vi "RandomLaser-1-1.vi"() -> ()   [LabVIEW 2014]
doc: "Random Laser Project\nAndré Romero - 2020\nandretec@ifsc.usp.br\n\nMain Program"
uses:
  OceanOptics.ctl
  GlobalVariables.vi
  <vilib>/Analysis/NI_AAL_SigProc.lvlib
  PowerMeterSteps.ctl
  <vilib>/Analysis/NI_AALBase.lvlib
  RL-Signal.ctl
  <vilib>/Utility/file.llb/Write To Spreadsheet File (DBL).vi
  <vilib>/Analysis/2dsp.llb/Integral Method.ctl
  <vilib>/Analysis/NI_AALPro.lvlib
  <vilib>/Analysis/8numeric.llb/1D Numeric Integration.vi
panel:
  out "Time Stamp":string="0:01:34"
  out "array of delay (ms)":u32[](array[numeric])=[842, 1108, 1021, 480, 726, 1312, 337, 999, 437, 1394, 1475, 822, 559, 616, 658, 1372, 991, 596, 810, 891, 815, 681, 1513, 577, 789, 631, 803, 488, 1470, 1213, 1450, 749, 1550, 888, 468, 582, 1321, 1466, 836, 595, 723, 733, 1457, 768, 669, 1441, 1356, 658, 1400, 1611, 522, 560, 750, 650, 906, 623, 657, 1594, 565, 802, 980, 736, 879, 514, 829, 685, 842, 615, 791, 1301, 1389, 1499, 389, 859, 1201, 1412, 555, 678, 866, 605, 785, 914, 554, 703, 796, 663, 608, 1407, 608, 816, 1001, 499, 881, 686, 1365, 829, 700, 715, 728, 1156, 922, 602, 1328, 1888]
  out "delta WL":dbl=0.38690207279938704
  in  "Stop":bool
  out "size(s)":i32=105
  out "Waveform Graph 2":dbl[](graph)=[-1.0602626e-05, -1.8573209307692306e-05, -1.2360805192307691e-05, -7.52886973076923e-06, 1.7781546653846153e-05, 2.90088355e-05, 7.443762192307693e-05, 0.00010577740999999999, 0.00011369514192307692, 0.0001716017673076923, 0.0001952365403846154, 0.00020954966423076922, 0.0002917340261538461, 0.00031620668153846155, 0.00033834876384615384, 0.00035088591038461535, 0.00036754105307692305, 0.0004927123461538461, 0.0005941180961538462, 0.0006408687538461539, 0.0007478033923076922, 0.0008147488615384615, 0.0008696404192307692, 0.0008872695615384616, 0.0009365023846153847, 0.001030977223076923, 0.0013047827038461537, 0.0015105027923076923, 0.0016743372076923077, 0.0017111218769230768, 0.0018390295192307693, 0.0019388902461538462, 0.0019474161, 0.0019474161, 0.001959032780769231, 0.0023469584115384614, 0.002392628811538462, 0.002490708273076923, 0.0025502076961538465, 0.0026105925461538462, 0.0027505951807692305, 0.0028934302884615383, 0.0031883340307692306, 0.003340183265384615, 0.003531661842307692, 0.003809862, 0.004016680999999999, 0.004217133384615384, 0.004234585384615385, 0.004321589269230769, 0.0046734980384615385, 0.0047475690769230765, 0.004773726692307693, 0.004844272115384615, 0.0048776663076923075, 0.004990282038461538, 0.005060921961538461, 0.005060921961538461, 0.0055383183461538464, 0.0056066344230769226, 0.0056979792692307685, 0.0058101301923076925, 0.006037626346153846, 0.006264335346153846, 0.006264335346153846, 0.006384484884615385, 0.006694922461538462, 0.006785941346153846, 0.006852017346153845, 0.007037507692307692, 0.007274539153846154, 0.007666755807692308, 0.007813228653846153, 0.007889473538461539, 0.007837736769230769, 0.007881207153846154, 0.007837807499999998, 0.007895348038461538, 0.008558267, 0.008670603307692306, 0.008750500961538461, 0.008750500961538461, 0.008761567576923077, 0.008665184615384614, 0.008665184615384614, 0.008836726192307692, 0.008947153307692307, 0.009076968, 0.0091185865, 0.009199394846153846, 0.009195958807692308, 0.009228286423076923, 0.009228286423076923, 0.009355492576923077, 0.009418467884615384, 0.009475817653846154, 0.009609611076923076, 0.009646632076923076, 0.009646632076923076, 0.009709267076923076, 0.009727449384615384, 0.009765767038461538, 0.009825513153846152, 0.009825513153846152, 0.009828276692307692]
  out "Motor Target":i32
  out "step error":dbl=4.630004747377598
  out "Numeric Control":i32=571
  out "appended array":dbl[](array[numeric])=[0.006088400884615384, 0.006019662115384615, 0.006051416192307692, 0.006051416192307692, 0.006124910076923076, 0.006172556192307692, 0.006457423115384615, 0.006457423115384615, 0.006727457423076923, 0.006873657153846154, 0.006931027961538462, 0.007085490076923076, 0.007085490076923076, 0.0074338476923076924, 0.0074338476923076924, 0.007682742307692307, 0.0077406902692307685, 0.007894204461538462, 0.008228431961538461, 0.008252353499999998, 0.008392664423076924, 0.008392664423076924, 0.00844546326923077, 0.008496700307692307, 0.008698614653846153, 0.008752471038461537, 0.008752471038461537, 0.008816909615384616, 0.008909836807692306, 0.009049831615384614, 0.009202393884615384, 0.009148910884615384, 0.009148910884615384, 0.00914061496153846, 0.009268187346153846, 0.009268187346153846, 0.009387016038461538, 0.009557217038461538, 0.009557217038461538, 0.009661707846153845, 0.009897883192307692, 0.009843781423076922, 0.010035894461538462, 0.010035894461538462, 0.010075476576923077, 0.009985933461538461, 0.009985933461538461, 0.010022820115384615, 0.009880154038461538, 0.009880154038461538, 0.009872941653846152, 0.009776705576923077, 0.009722396961538461, 0.009722396961538461, 0.00970868323076923, 0.009762843192307693, 0.009601696653846154, 0.009404687, 0.009404687, 0.009369634346153845, 0.009404875038461538, 0.009404875038461538, 0.009498904615384616, 0.009371503269230768, 0.00918766646153846, 0.009124002499999999, 0.009124002499999999, 0.008958641692307694, 0.008990724846153847, 0.00885226673076923, 0.008834460576923076, 0.008834460576923076, 0.008653751769230769, 0.00856737246153846, 0.00856737246153846, 0.008425105807692308, 0.008425105807692308, 0.008219209192307692, 0.008219209192307692, 0.00784359423076923, 0.00784359423076923, 0.007704991961538461, 0.007290269076923077, 0.007167071692307693, 0.007167071692307693, 0.007004637807692307, 0.006663415999999999, 0.006663415999999999, 0.006437745346153846, 0.006437745346153846, 0.006332175461538462, 0.006191508153846154, 0.005999933307692308, 0.005999933307692308, 0.005755351423076923, 0.005602332884615384, 0.005341360192307692, 0.005145278269230769, 0.005095772230769231, 0.005095772230769231, 0.004993629423076923, 0.004931614538461538, 0.004852756999999999, 0.0045647115, 0.004118548884615384, 0.004118548884615384, 0.0038448551038461534, 0.0038448551038461534, 0.0036742806846153846, 0.0035786020692307693, 0.0034039533384615387, 0.003279750280769231, 0.0031362856346153845, 0.002992311446153846, 0.00278225455, 0.00278225455, 0.0027080816499999998, 0.0023620212076923075, 0.0023620212076923075, 0.0022386317153846153, 0.002112930703846154, 0.001966992230769231, 0.001864995396153846, 0.0016025416423076924, 0.0015336607115384615, 0.0015336607115384615, 0.00138643115, 0.001199871676923077, 0.001054965946153846, 0.0009808228153846154, 0.0009352345230769231, 0.0009352345230769231, 0.0008112675961538462, 0.0007670655923076923, 0.0006205916653846153, 0.0005729669423076923, 0.0004712719461538462, 0.0004253776961538461, 0.00037583648423076925, 0.0003179948042307692, 0.0003179948042307692, 0.00023497789076923074, 0.00016738367076923075, 0.00010301030038461539, 0.00010301030038461539, -5.387276884615384e-06, -1.463806623076923e-05, -1.463806623076923e-05, -4.7211138846153846e-05, -6.807878461538462e-05, -6.807878461538462e-05, -7.410832192307692e-05, -7.496382769230768e-05, -7.496382769230768e-05, -7.545941807692307e-05, -5.749450153846154e-05, -5.749450153846154e-05, -3.4196017846153845e-05, -3.935870692307692e-06, 1.5409708653846153e-05, 1.5409708653846153e-05, 6.494484076923077e-05, 0.00010907543384615385, 0.00018819801653846153, 0.00018819801653846153, 0.0002518573846153846, 0.0002518573846153846, 0.00036352903423076923, 0.00036352903423076923, 0.00041147177307692307, 0.0006472696384615385, 0.0007086754153846153, 0.0007086754153846153, 0.0008853873846153846, 0.0008853873846153846, 0.0010021450653846153, 0.0011826555307692308, 0.0011826555307692308, 0.0012722923076923078, 0.0014195047423076923, 0.0014195047423076923, 0.001521211773076923, 0.0019048786115384614, 0.0019904611115384614, 0.0019904611115384614, 0.0022153737230769226, 0.002316673857692308, 0.0024764594846153846, 0.002645395580769231, 0.002645395580769231, 0.0027565079615384618, 0.0028778550384615386, 0.0029616142961538462, 0.0030646022269230767, 0.0033371978846153845, 0.0036325316884615387, 0.003766581919230769, 0.0038838421538461535, 0.004069579192307693, 0.004069579192307693, 0.004217383230769231, 0.004395655846153846, 0.004597885384615385, 0.004702704384615384, 0.005098710807692307, 0.005098710807692307, 0.005233906153846154, 0.005420664076923077, 0.005420664076923077, 0.005705798807692308, 0.005807721769230769, 0.005997826192307692, 0.005997826192307692, 0.006048182961538462, 0.006420420961538461, 0.006442509, 0.006442509, 0.006588312, 0.006697340769230769, 0.0068355065, 0.007070677538461538, 0.007342427192307692, 0.007342427192307692, 0.007521121115384615, 0.0075672636923076915, 0.0075672636923076915, 0.007820148192307693, 0.007926758653846153, 0.008071146807692308, 0.008098770346153847, 0.008098770346153847, 0.008299234846153846, 0.008456086615384615, 0.008540288884615384, 0.008588171423076923, 0.008658632230769231, 0.008842661576923077, 0.008987104346153846, 0.009063884730769231, 0.009099668115384615, 0.009163529076923077, 0.009163529076923077, 0.009278776653846153, 0.00929891473076923, 0.009298505461538462, 0.009352490846153846, 0.009341272000000001, 0.009346393384615384, 0.009460399769230769, 0.009600639961538461, 0.009552550576923077, 0.009686249999999999, 0.009748534884615384, 0.009748534884615384, 0.009754034153846153, 0.009697521692307691, 0.009786861499999999, 0.009818387653846154, 0.009818387653846154, 0.009936413961538462, 0.009839843884615385, 0.009827076692307693, 0.009686187307692308, 0.009518681769230769, 0.009597393769230769, 0.009587433076923077, 0.009642559307692306, 0.009593832346153845, 0.009555409, 0.009555409, 0.009464713423076922, 0.00935705523076923, 0.009246092615384616, 0.009100211692307692, 0.008999765846153846, 0.009005339461538461, 0.00912219803846154, 0.009071167846153846, 0.00880848026923077, 0.008668077115384617, 0.00842139573076923, 0.008434145, 0.00836997776923077, 0.008148135846153846, 0.0079498895, 0.007826445384615384, 0.007592567884615384, 0.007468364384615384, 0.007434496923076923, 0.007345466961538461, 0.0072643729615384615, 0.007099095884615384, 0.006919479576923077, 0.0067396438846153844, 0.006546222961538461, 0.006338919499999999, 0.006158986615384615, 0.0060612904615384615, 0.006015968615384616, 0.006006780769230769, 0.0057571594615384615, 0.005552136384615384, 0.005526767269230769, 0.005398911, 0.005002913961538461, 0.004812826576923077, 0.0045138299230769235, 0.004511429538461538, 0.004511429538461538, 0.00449410023076923, 0.0041596291538461535, 0.003989496653846154, 0.003923653961538461, 0.0038588970384615382, 0.00366277415, 0.00366277415, 0.003438994126923077, 0.003438994126923077, 0.0033308669038461538, 0.002999190473076923, 0.002931602423076923, 0.002931602423076923, 0.0028267784884615384, 0.0024557568115384613, 0.0024557568115384613, 0.0023362327538461536, 0.0020663858423076924, 0.001972159503846154, 0.001749807696153846, 0.0017157880038461539, 0.0014433754807692306, 0.0013448947230769231, 0.0013372903384615386, 0.001248845923076923, 0.0010909017884615383, 0.0009248163, 0.0007581637961538461, 0.000743720346153846, 0.00072130105, 0.0006646627576923077, 0.0005633626769230768, 0.0005633626769230768, 0.0004006925538461538, 0.0003739367319230769, 0.00025180435423076923, 0.0002452021223076923, 0.00022705456884615383, 0.00016810932153846155, 8.971818923076923e-05, 7.203049038461537e-05, 6.765868923076923e-05, 4.472013076923077e-05, 1.969299146153846e-05, 5.592379307692308e-06, 5.232428384615384e-06, 2.3887723115384613e-06, -7.4403199230769226e-06, -1.0602626e-05, -1.8573209307692306e-05, -1.2360805192307691e-05, -7.52886973076923e-06, 1.7781546653846153e-05, 2.90088355e-05, 7.443762192307693e-05, 0.00010577740999999999, 0.00011369514192307692, 0.0001716017673076923, 0.0001952365403846154, 0.00020954966423076922, 0.0002917340261538461, 0.00031620668153846155, 0.00033834876384615384, 0.00035088591038461535, 0.00036754105307692305, 0.0004927123461538461, 0.0005941180961538462, 0.0006408687538461539, 0.0007478033923076922, 0.0008147488615384615, 0.0008696404192307692, 0.0008872695615384616, 0.0009365023846153847, 0.001030977223076923, 0.0013047827038461537, 0.0015105027923076923, 0.0016743372076923077, 0.0017111218769230768, 0.0018390295192307693, 0.0019388902461538462, 0.0019474161, 0.0019474161, 0.001959032780769231, 0.0023469584115384614, 0.002392628811538462, 0.002490708273076923, 0.0025502076961538465, 0.0026105925461538462, 0.0027505951807692305, 0.0028934302884615383, 0.0031883340307692306, 0.003340183265384615, 0.003531661842307692, 0.003809862, 0.004016680999999999, 0.004217133384615384, 0.004234585384615385, 0.004321589269230769, 0.0046734980384615385, 0.0047475690769230765, 0.004773726692307693, 0.004844272115384615, 0.0048776663076923075, 0.004990282038461538, 0.005060921961538461, 0.005060921961538461, 0.0055383183461538464, 0.0056066344230769226, 0.0056979792692307685, 0.0058101301923076925, 0.006037626346153846, 0.006264335346153846, 0.006264335346153846, 0.006384484884615385, 0.006694922461538462, 0.006785941346153846, 0.006852017346153845, 0.007037507692307692, 0.007274539153846154, 0.007666755807692308, 0.007813228653846153, 0.007889473538461539, 0.007837736769230769, 0.007881207153846154, 0.007837807499999998, 0.007895348038461538, 0.008558267, 0.008670603307692306, 0.008750500961538461, 0.008750500961538461, 0.008761567576923077, 0.008665184615384614, 0.008665184615384614, 0.008836726192307692, 0.008947153307692307, 0.009076968, 0.0091185865, 0.009199394846153846, 0.009195958807692308, 0.009228286423076923, 0.009228286423076923, 0.009355492576923077, 0.009418467884615384, 0.009475817653846154, 0.009609611076923076, 0.009646632076923076, 0.009646632076923076, 0.009709267076923076, 0.009727449384615384, 0.009765767038461538, 0.009825513153846152, 0.009825513153846152, 0.009828276692307692, 0.009801360576923077, 0.009814088346153845, 0.00984271126923077, 0.009860809384615385, 0.009873510307692308, 0.0098137955, 0.009603421384615384, 0.009603421384615384, 0.00955146523076923, 0.00949282146153846, 0.009467082038461538, 0.009361033923076922, 0.00934043826923077, 0.009350373884615385, 0.009290900884615384, 0.009237378461538461, 0.009179430499999999, 0.00911498746153846, 0.009004738576923075, 0.008925467807692307, 0.008768998461538462, 0.008696039153846154, 0.008603960038461539, 0.008526891307692307, 0.008526891307692307, 0.008431125346153846, 0.008406236653846154, 0.008305084269230769, 0.008305084269230769, 0.007906728076923077, 0.007751959269230769, 0.007706900269230769, 0.0076030416923076926, 0.007524473884615385, 0.007239447076923077, 0.007210126076923076, 0.00707238573076923, 0.006996408615384615, 0.006782788269230768, 0.006661043807692307, 0.006556346153846154, 0.006556346153846154, 0.006124177538461538, 0.006010642153846154, 0.005964971538461539, 0.005829333346153846, 0.005684320153846154, 0.005567964846153846, 0.005567964846153846, 0.005230584730769231, 0.005230584730769231, 0.00491325, 0.004761246499999999, 0.0046623946923076915, 0.004590434807692308, 0.004465162961538461, 0.004297437115384615, 0.004162477307692308, 0.004078199769230769, 0.003986143884615385, 0.0038567899230769233, 0.0035312552846153847, 0.003443240823076923, 0.003361292719230769, 0.0032899939346153844, 0.0032048941076923076, 0.0030188552615384614, 0.0029103387192307693, 0.0027534209384615384, 0.0025445671499999996, 0.0024274378884615385, 0.0022463663923076925, 0.002153195626923077, 0.002153195626923077, 0.001970726030769231, 0.0015185043307692307, 0.0014648517576923076, 0.00142660865, 0.0013723234038461537, 0.0013325882807692308, 0.0011872456538461538, 0.0011872456538461538, 0.0009419369653846152, 0.0009419369653846152, 0.0007446580500000001, 0.0005823951846153846, 0.0005605902038461537, 0.0005284770346153846, 0.00048518973461538455, 0.0003851460153846154, 0.00034837271076923075, 0.00029723269115384615, 0.00029723269115384615, 0.0001553477396153846, 0.0001553477396153846, 0.00010404294076923076, 4.2784963846153846e-05, 4.2784963846153846e-05, -7.568358769230769e-05, -8.80733123076923e-05, -8.80733123076923e-05, -0.00011827445499999998, -0.00014029274807692306, -0.00014605101076923076, -0.00014586807653846153, -0.00014213945615384614, -0.00014143732615384615, -0.00013074085692307692, -0.00010745426653846153, -8.991409423076923e-05]
  out "Locations":dbl[](array[numeric])=[152.05783514633893, 357.0837553051094, 566.3699952526224]
  out "Amplitudes":dbl[](array[numeric])=[-7.71015385680156e-05, -1.3525658190277859e-05, -0.0001490156983661843]
  out "standard deviation":dbl=3.0125010126431166 format="%0.2f"
  out "mean":dbl=207.15608005314175 format="%0.2f"
  out "Array":dbl[](array[numeric])=[205.02592015877045, 209.28623994751302]
  out "# found":i32=3
  in  "Select Light Source":u16(ring)=6
  in  "Tab Control":T1(tab)=enum."Aquisition"
  out "Current Step":dbl=103.0
  out "Running":bool=TRUE
  in  "Range List":T2(array[cluster])=[{"Name"="Sample", "Inicial"=500.0, "Final"=700.0}]
  out "Current Position":dbl=104.0
  out "Min power to Aqc":dbl
  out "Max power to Aqc":dbl
  out "Low power":bool
  out "Max power":bool
  in  "Clear Dark Spec":bool caption="Blank Button"
  in  "Average":i32=5
  in  "Integration Time":i32=100
  out "Spectrum":T3(graph)
  in  "Store Dark Spec":bool caption="Blank Button"
  in  "threshold":dbl=300.0 format="%0.2f"
  in  "width":i32=20 min=3
  out "Power Meter [W]":dbl=0.03652572625 format="%#_4p"
  in  "Power up":bool
  in  "Power down":bool
  in  "Half Power":bool
  in  "min Power":bool
  in  "max Power Go":bool
  out "Max Power":dbl=0.010075476576923077 format="%#_3p"
  out "Min Power":dbl=-0.00014605101076923076 format="%#_3p"
  in  "Correct Electrical Dark":bool
  out "table":string[][](table)=[["Name", "FWHM", "Peak", "WL"], ["Sample", "283", "0", "0.00"]]
  out "FWHM":dbl=283.41913100133013 format="%#_4g"
  out "Power Meter":dbl=0.03652572625 format="%#_4p"
  in  "Tuning Motor":bool
  out "Power Meter":dbl(graph)=-8.991409423076923e-05
  out "Min Power":dbl=-0.00014605101076923076 format="%#_3p"
  out "Max Power":dbl=0.010075476576923077 format="%#_3p"
  out "threshold":dbl=0.004964712783076923
  out "Motor Steps Max":i32=104
  out "peak":cluster{dbl[], dbl[]}(graph)={[0.0005015534046874999, 0.0004468511640625, 0.00042210990624999995, 0.0004196072953125, 0.0004832955703125, 0.00061629739375, 0.0006558638234375, 0.0007916550203125, 0.0008665692796875, 0.0009977359703125, 0.0011809348499999999, 0.0014192177328125, 0.0014146657125, 0.001802492625, 0.001933848765625, 0.002189746375, 0.002470051546875, 0.0026339437656249997, 0.002995718203125, 0.0031850202499999996, 0.003397749609375, 0.0038501235468749997, 0.00424369390625, 0.004263668234375, 0.00491242171875, 0.005129561390625001, 0.005458205125, 0.005549518390625, 0.0062437480625, 0.00666187115625, 0.0070897651249999995, 0.007395214921875, 0.00802906796875, 0.008537028765625, 0.00851176228125, 0.008568135671875001, 0.009842375578125, 0.010231534546875, 0.010585043484374999, 0.011054932109375, 0.011588129562499999, 0.012016717671875, 0.0123040546875, 0.013023524656249999, 0.013643318375000001, 0.014436681515624999, 0.01473497978125, 0.014904356796875, 0.0159008428125, 0.016111576406249998, 0.0166677578125, 0.01671055796875, 0.01781797625, 0.018240680156249998, 0.0187542390625, 0.019142343125, 0.0198526453125, 0.01996271609375, 0.02116104, 0.0210028971875, 0.022299682343750002, 0.022769914375000002, 0.02304846125, 0.0231955665625, 0.023897850781249997, 0.024010065, 0.02472973140625, 0.02519956328125, 0.025853811562500002, 0.026471383125, 0.026681425468750002, 0.02802214578125, 0.0278189225, 0.02824113765625, 0.02908268078125, 0.0292354059375, 0.030335440468750002, 0.030317477656249998, 0.03099246828125, 0.03051971140625, 0.031873135625, 0.031079078281250002, 0.032200833125, 0.03170667328125, 0.031286408125, 0.0332111609375, 0.03241316296875, 0.03332632484375, 0.03400264828125, 0.0332313328125, 0.033794730625, 0.03382630828125, 0.03476316046875, 0.034105763125, 0.0363623665625, 0.0356505421875, 0.03637592890625, 0.03534870921875, 0.034879485625, 0.03543325, 0.03644525421875, 0.0360509496875, 0.03622908546875, 0.0367265165625], [0.0, 0.0, 0.0, 0.0, 0.0, 0.0, 0.0, 0.0, 0.0, 0.0, 394.1588118886737, 394.1588118886737, 431.6253969371716, 498.6580958932715, 726.8856416219951, 730.4930041074641, 924.368639084171, 924.368639084171, 1127.8876724584377, 1176.6893948954707, 1257.9781408404046, 1467.6796179824566, 1607.7224288634548, 1607.7224288634548, 1680.7493036733524, 2162.6044383453827, 2162.6044383453827, 2448.692515986958, 2958.1440153813733, 3289.2072493799756, 3712.6227202169744, 3916.1593851910925, 4488.731356999813, 4745.2298607199955, 4745.2298607199955, 5198.759914364481, 6270.088662889236, 6752.182794036469, 6752.182794036469, 7804.8560091986965, 7277.151040936606, 8792.865300035679, 9705.844619862504, 10118.9500660173, 10697.214391856975, 11484.64595778735, 12094.126688665461, 11954.607877343742, 13538.141020872097, 13237.333536906832, 13237.333536906832, 14090.070182374848, 14076.663576921685, 16519.70865370654, 17067.47933725341, 17301.50532254216, 18483.407890232967, 19382.85944297429, 20252.918803668017, 20252.918803668017, 21897.31684455097, 21881.77133506106, 22939.78950340062, 22939.78950340062, 24400.94207257171, 24400.94207257171, 21943.9132770401, 25836.512442775784, 26753.422445361583, 28622.125850531873, 28566.341648867947, 30696.155691767697, 30696.155691767697, 31037.50720247306, 31952.22245683209, 31579.102102413905, 31579.102102413905, 33472.21756510413, 35005.5223676299, 35573.41340181915, 35750.55108838855, 35924.52495802316, 35751.327930291336, 35751.327930291336, 35440.30537928901, 37586.25874441115, 37883.715024127945, 40728.053135189504, 40728.053135189504, 38884.561951946256, 39029.25713331435, 39029.25713331435, 39436.46265344174, 41071.4281739883, 43284.48665620081, 43284.48665620081, 42497.26030199413, 41645.324274929924, 40896.30949743132, 42085.672828850686, 42085.672828850686, 44605.47818116084, 44668.345249601494, 43659.80224543728]}
  out "peak Log":cluster{dbl[], dbl[]}(graph)={[0.0005015534046874999, 0.0004468511640625, 0.00042210990624999995, 0.0004196072953125, 0.0004832955703125, 0.00061629739375, 0.0006558638234375, 0.0007916550203125, 0.0008665692796875, 0.0009977359703125, 0.0011809348499999999, 0.0014192177328125, 0.0014146657125, 0.001802492625, 0.001933848765625, 0.002189746375, 0.002470051546875, 0.0026339437656249997, 0.002995718203125, 0.0031850202499999996, 0.003397749609375, 0.0038501235468749997, 0.00424369390625, 0.004263668234375, 0.00491242171875, 0.005129561390625001, 0.005458205125, 0.005549518390625, 0.0062437480625, 0.00666187115625, 0.0070897651249999995, 0.007395214921875, 0.00802906796875, 0.008537028765625, 0.00851176228125, 0.008568135671875001, 0.009842375578125, 0.010231534546875, 0.010585043484374999, 0.011054932109375, 0.011588129562499999, 0.012016717671875, 0.0123040546875, 0.013023524656249999, 0.013643318375000001, 0.014436681515624999, 0.01473497978125, 0.014904356796875, 0.0159008428125, 0.016111576406249998, 0.0166677578125, 0.01671055796875, 0.01781797625, 0.018240680156249998, 0.0187542390625, 0.019142343125, 0.0198526453125, 0.01996271609375, 0.02116104, 0.0210028971875, 0.022299682343750002, 0.022769914375000002, 0.02304846125, 0.0231955665625, 0.023897850781249997, 0.024010065, 0.02472973140625, 0.02519956328125, 0.025853811562500002, 0.026471383125, 0.026681425468750002, 0.02802214578125, 0.0278189225, 0.02824113765625, 0.02908268078125, 0.0292354059375, 0.030335440468750002, 0.030317477656249998, 0.03099246828125, 0.03051971140625, 0.031873135625, 0.031079078281250002, 0.032200833125, 0.03170667328125, 0.031286408125, 0.0332111609375, 0.03241316296875, 0.03332632484375, 0.03400264828125, 0.0332313328125, 0.033794730625, 0.03382630828125, 0.03476316046875, 0.034105763125, 0.0363623665625, 0.0356505421875, 0.03637592890625, 0.03534870921875, 0.034879485625, 0.03543325, 0.03644525421875, 0.0360509496875, 0.03622908546875, 0.0367265165625], [0.0, 0.0, 0.0, 0.0, 0.0, 0.0, 0.0, 0.0, 0.0, 0.0, 394.1588118886737, 394.1588118886737, 431.6253969371716, 498.6580958932715, 726.8856416219951, 730.4930041074641, 924.368639084171, 924.368639084171, 1127.8876724584377, 1176.6893948954707, 1257.9781408404046, 1467.6796179824566, 1607.7224288634548, 1607.7224288634548, 1680.7493036733524, 2162.6044383453827, 2162.6044383453827, 2448.692515986958, 2958.1440153813733, 3289.2072493799756, 3712.6227202169744, 3916.1593851910925, 4488.731356999813, 4745.2298607199955, 4745.2298607199955, 5198.759914364481, 6270.088662889236, 6752.182794036469, 6752.182794036469, 7804.8560091986965, 7277.151040936606, 8792.865300035679, 9705.844619862504, 10118.9500660173, 10697.214391856975, 11484.64595778735, 12094.126688665461, 11954.607877343742, 13538.141020872097, 13237.333536906832, 13237.333536906832, 14090.070182374848, 14076.663576921685, 16519.70865370654, 17067.47933725341, 17301.50532254216, 18483.407890232967, 19382.85944297429, 20252.918803668017, 20252.918803668017, 21897.31684455097, 21881.77133506106, 22939.78950340062, 22939.78950340062, 24400.94207257171, 24400.94207257171, 21943.9132770401, 25836.512442775784, 26753.422445361583, 28622.125850531873, 28566.341648867947, 30696.155691767697, 30696.155691767697, 31037.50720247306, 31952.22245683209, 31579.102102413905, 31579.102102413905, 33472.21756510413, 35005.5223676299, 35573.41340181915, 35750.55108838855, 35924.52495802316, 35751.327930291336, 35751.327930291336, 35440.30537928901, 37586.25874441115, 37883.715024127945, 40728.053135189504, 40728.053135189504, 38884.561951946256, 39029.25713331435, 39029.25713331435, 39436.46265344174, 41071.4281739883, 43284.48665620081, 43284.48665620081, 42497.26030199413, 41645.324274929924, 40896.30949743132, 42085.672828850686, 42085.672828850686, 44605.47818116084, 44668.345249601494, 43659.80224543728]}
  out "FWHM":cluster{dbl[], dbl[]}(graph)={[0.0005015534046874999, 0.0004468511640625, 0.00042210990624999995, 0.0004196072953125, 0.0004832955703125, 0.00061629739375, 0.0006558638234375, 0.0007916550203125, 0.0008665692796875, 0.0009977359703125, 0.0011809348499999999, 0.0014192177328125, 0.0014146657125, 0.001802492625, 0.001933848765625, 0.002189746375, 0.002470051546875, 0.0026339437656249997, 0.002995718203125, 0.0031850202499999996, 0.003397749609375, 0.0038501235468749997, 0.00424369390625, 0.004263668234375, 0.00491242171875, 0.005129561390625001, 0.005458205125, 0.005549518390625, 0.0062437480625, 0.00666187115625, 0.0070897651249999995, 0.007395214921875, 0.00802906796875, 0.008537028765625, 0.00851176228125, 0.008568135671875001, 0.009842375578125, 0.010231534546875, 0.010585043484374999, 0.011054932109375, 0.011588129562499999, 0.012016717671875, 0.0123040546875, 0.013023524656249999, 0.013643318375000001, 0.014436681515624999, 0.01473497978125, 0.014904356796875, 0.0159008428125, 0.016111576406249998, 0.0166677578125, 0.01671055796875, 0.01781797625, 0.018240680156249998, 0.0187542390625, 0.019142343125, 0.0198526453125, 0.01996271609375, 0.02116104, 0.0210028971875, 0.022299682343750002, 0.022769914375000002, 0.02304846125, 0.0231955665625, 0.023897850781249997, 0.024010065, 0.02472973140625, 0.02519956328125, 0.025853811562500002, 0.026471383125, 0.026681425468750002, 0.02802214578125, 0.0278189225, 0.02824113765625, 0.02908268078125, 0.0292354059375, 0.030335440468750002, 0.030317477656249998, 0.03099246828125, 0.03051971140625, 0.031873135625, 0.031079078281250002, 0.032200833125, 0.03170667328125, 0.031286408125, 0.0332111609375, 0.03241316296875, 0.03332632484375, 0.03400264828125, 0.0332313328125, 0.033794730625, 0.03382630828125, 0.03476316046875, 0.034105763125, 0.0363623665625, 0.0356505421875, 0.03637592890625, 0.03534870921875, 0.034879485625, 0.03543325, 0.03644525421875, 0.0360509496875, 0.03622908546875, 0.0367265165625], [397.83240728192527, 415.17504165662353, 426.25368524810295, 426.25368524810295, 206.73115418767736, 463.69050128006853, 463.69050128006853, 20.243933101369635, 20.243933101369635, 17.116594601847964, 20.241392797112326, 20.241392797112326, 28.609780989435308, 26.179034684086332, 28.5989916901716, 28.949572169655312, 31.723831233679903, 31.723831233679903, 30.6722195921933, 31.723831233679903, 29.98647772865229, 29.632206705867475, 28.588191211899016, 28.588191211899016, 29.28175605364379, 27.533626517494895, 27.533626517494895, 25.442507029580838, 23.695414233195834, 20.560596555511665, 18.812252502514298, 18.462714458332698, 15.671948237431252, 16.368473811981517, 16.368473811981517, 15.322715880405667, 13.578930006455039, 13.578930006455039, 13.578930006455039, 12.882578171121622, 12.533608422419206, 12.533608422419206, 11.488417756278523, 11.488417756278523, 11.488417756278523, 11.488417756278523, 11.140990757941722, 10.792152517895033, 10.792152517895033, 10.792152517895033, 10.792152517895033, 10.792152517895033, 10.792152517895033, 10.095886809932495, 10.095886809932495, 10.443358144362264, 9.74713631806128, 9.74713631806128, 9.74713631806128, 9.74713631806128, 9.74713631806128, 10.095886809932495, 9.74713631806128, 9.74713631806128, 9.74713631806128, 9.74713631806128, 9.74713631806128, 9.74713631806128, 9.398429722999595, 9.050914067624603, 9.398429722999595, 9.399620662686289, 9.399620662686289, 9.74713631806128, 9.74713631806128, 9.74713631806128, 9.74713631806128, 9.398429722999595, 9.050914067624603, 9.050914067624603, 9.050914067624603, 9.399620662686289, 9.74713631806128, 9.74713631806128, 8.702251384519855, 9.398429722999595, 9.398429722999595, 9.050914067624603, 9.050914067624603, 9.050914067624603, 9.050914067624603, 9.050914067624603, 9.74713631806128, 9.399620662686289, 9.399620662686289, 9.399620662686289, 9.050914067624603, 9.050914067624603, 9.050914067624603, 9.399620662686289, 9.399620662686289, 9.050914067624603, 9.050914067624603, 9.74713631806128]}
  in  "File name":string="N28-TiO2-30uL-2"
  out "Current Step":dbl=104.0
  out "Power Meter [W]":dbl=0.03652572625 format="%#_4p"
  out "Running":bool
  in  "Step Stop":i32=104
  in  "Save Aquisition":bool
  in  "Play Aquisition":bool
  out "Integration":cluster{dbl[], dbl[]}(graph)={[0.0005015534046874999, 0.0004468511640625, 0.00042210990624999995, 0.0004196072953125, 0.0004832955703125, 0.00061629739375, 0.0006558638234375, 0.0007916550203125, 0.0008665692796875, 0.0009977359703125, 0.0011809348499999999, 0.0014192177328125, 0.0014146657125, 0.001802492625, 0.001933848765625, 0.002189746375, 0.002470051546875, 0.0026339437656249997, 0.002995718203125, 0.0031850202499999996, 0.003397749609375, 0.0038501235468749997, 0.00424369390625, 0.004263668234375, 0.00491242171875, 0.005129561390625001, 0.005458205125, 0.005549518390625, 0.0062437480625, 0.00666187115625, 0.0070897651249999995, 0.007395214921875, 0.00802906796875, 0.008537028765625, 0.00851176228125, 0.008568135671875001, 0.009842375578125, 0.010231534546875, 0.010585043484374999, 0.011054932109375, 0.011588129562499999, 0.012016717671875, 0.0123040546875, 0.013023524656249999, 0.013643318375000001, 0.014436681515624999, 0.01473497978125, 0.014904356796875, 0.0159008428125, 0.016111576406249998, 0.0166677578125, 0.01671055796875, 0.01781797625, 0.018240680156249998, 0.0187542390625, 0.019142343125, 0.0198526453125, 0.01996271609375, 0.02116104, 0.0210028971875, 0.022299682343750002, 0.022769914375000002, 0.02304846125, 0.0231955665625, 0.023897850781249997, 0.024010065, 0.02472973140625, 0.02519956328125, 0.025853811562500002, 0.026471383125, 0.026681425468750002, 0.02802214578125, 0.0278189225, 0.02824113765625, 0.02908268078125, 0.0292354059375, 0.030335440468750002, 0.030317477656249998, 0.03099246828125, 0.03051971140625, 0.031873135625, 0.031079078281250002, 0.032200833125, 0.03170667328125, 0.031286408125, 0.0332111609375, 0.03241316296875, 0.03332632484375, 0.03400264828125, 0.0332313328125, 0.033794730625, 0.03382630828125, 0.03476316046875, 0.034105763125, 0.0363623665625, 0.0356505421875, 0.03637592890625, 0.03534870921875, 0.034879485625, 0.03543325, 0.03644525421875, 0.0360509496875, 0.03622908546875, 0.0367265165625], [0.0, 0.0, 0.0, 0.0, 0.0, 0.0, 0.0, 0.0, 0.0, 0.0, 394.1588118886737, 394.1588118886737, 431.6253969371716, 498.6580958932715, 726.8856416219951, 730.4930041074641, 924.368639084171, 924.368639084171, 1127.8876724584377, 1176.6893948954707, 1257.9781408404046, 1467.6796179824566, 1607.7224288634548, 1607.7224288634548, 1680.7493036733524, 2162.6044383453827, 2162.6044383453827, 2448.692515986958, 2958.1440153813733, 3289.2072493799756, 3712.6227202169744, 3916.1593851910925, 4488.731356999813, 4745.2298607199955, 4745.2298607199955, 5198.759914364481, 6270.088662889236, 6752.182794036469, 6752.182794036469, 7804.8560091986965, 7277.151040936606, 8792.865300035679, 9705.844619862504, 10118.9500660173, 10697.214391856975, 11484.64595778735, 12094.126688665461, 11954.607877343742, 13538.141020872097, 13237.333536906832, 13237.333536906832, 14090.070182374848, 14076.663576921685, 16519.70865370654, 17067.47933725341, 17301.50532254216, 18483.407890232967, 19382.85944297429, 20252.918803668017, 20252.918803668017, 21897.31684455097, 21881.77133506106, 22939.78950340062, 22939.78950340062, 24400.94207257171, 24400.94207257171, 21943.9132770401, 25836.512442775784, 26753.422445361583, 28622.125850531873, 28566.341648867947, 30696.155691767697, 30696.155691767697, 31037.50720247306, 31952.22245683209, 31579.102102413905, 31579.102102413905, 33472.21756510413, 35005.5223676299, 35573.41340181915, 35750.55108838855, 35924.52495802316, 35751.327930291336, 35751.327930291336, 35440.30537928901, 37586.25874441115, 37883.715024127945, 40728.053135189504, 40728.053135189504, 38884.561951946256, 39029.25713331435, 39029.25713331435, 39436.46265344174, 41071.4281739883, 43284.48665620081, 43284.48665620081, 42497.26030199413, 41645.324274929924, 40896.30949743132, 42085.672828850686, 42085.672828850686, 44605.47818116084, 44668.345249601494, 43659.80224543728]}
  in  "correction factor":dbl=0.64
  out "Power Value":dbl=0.03652572625 caption="Optical Power [W]" format="%#_4p"
  in  "Average Time (0.0)":dbl=0.05
  out "P Meter Delay (ms)":u32=106
  out "Spectrum delay (ms)":u32=707
  out "Delayreturn":u32
  # "Set power to Aquisition"
  # "Move Step Motor"
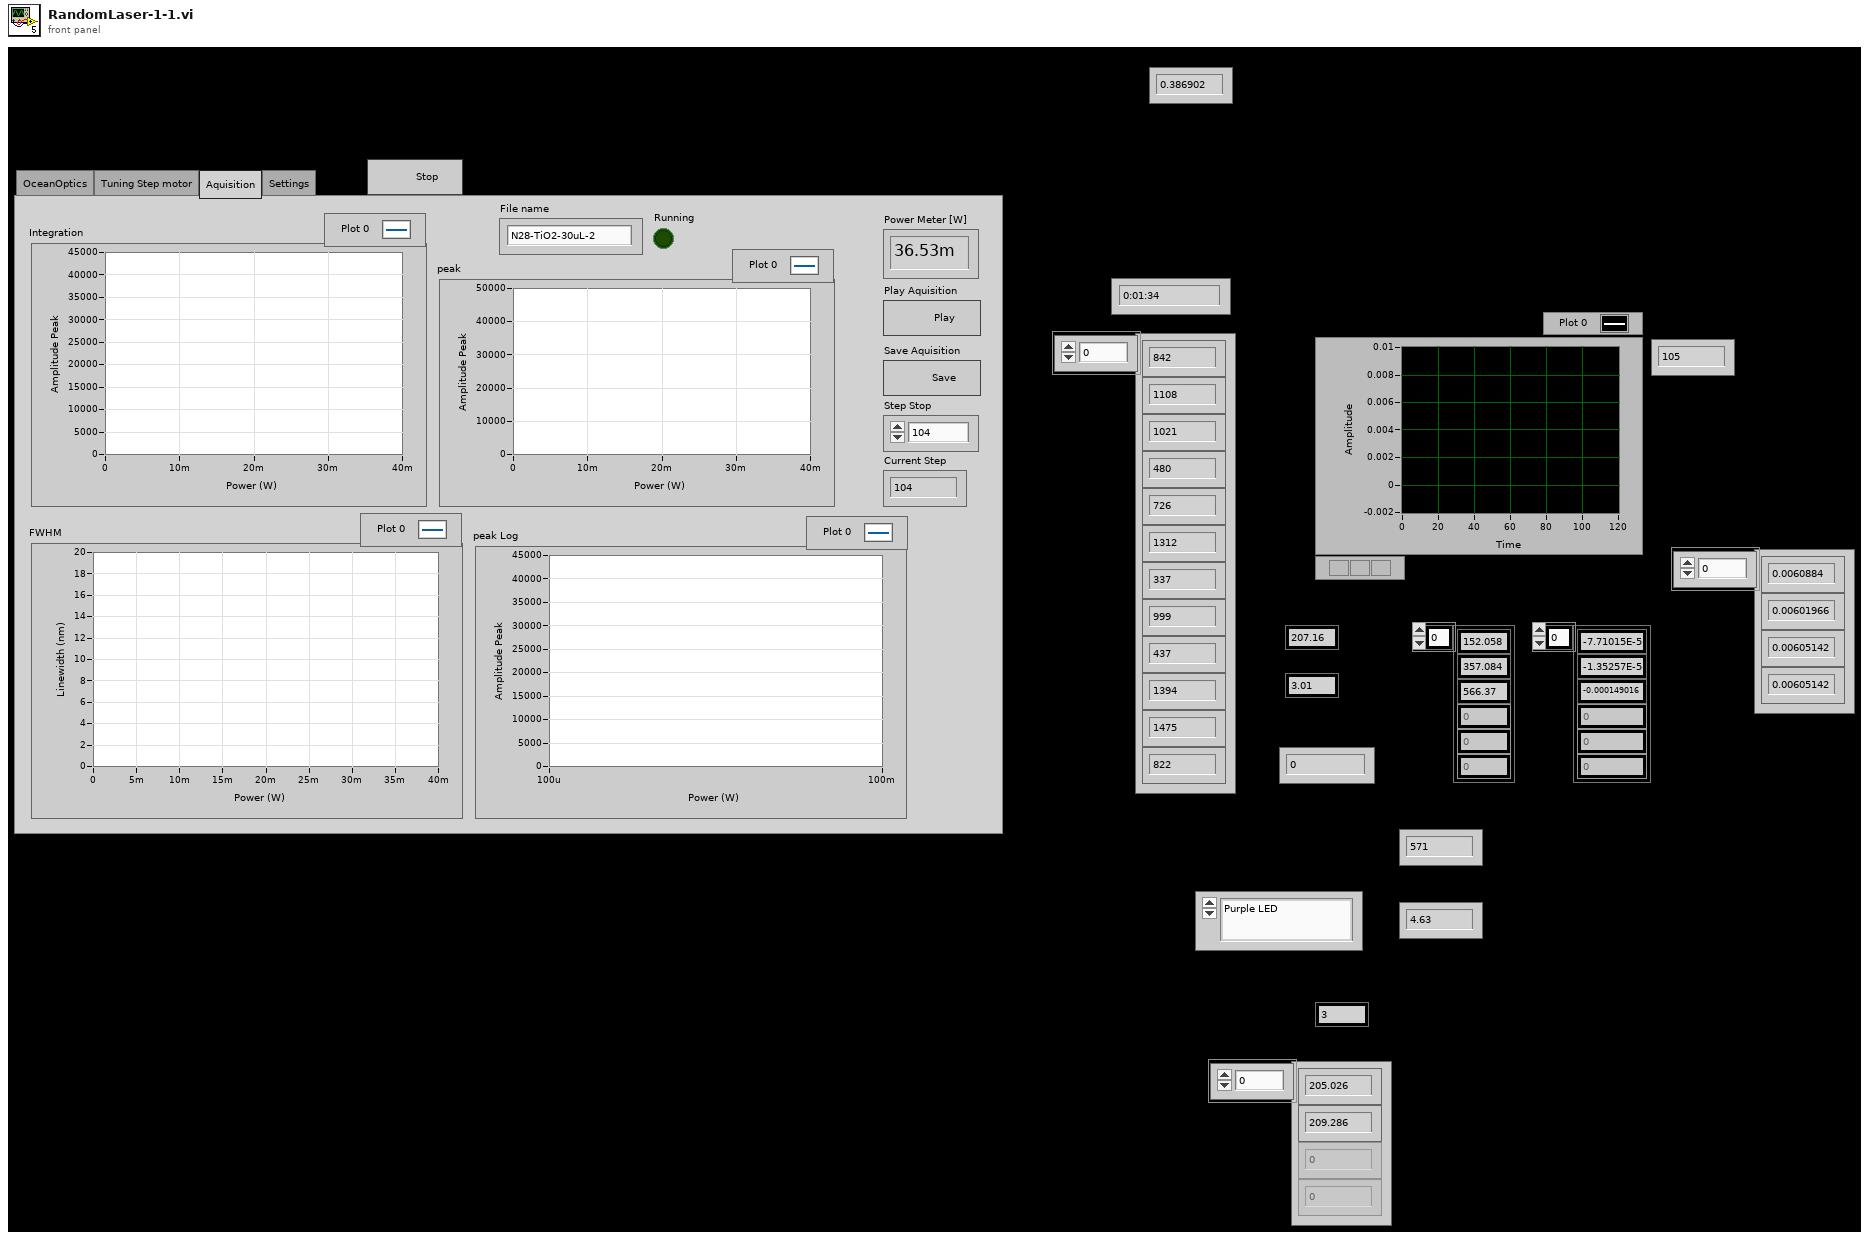
[diagram p1: front panel]
types:
  T1 = enum32{"OceanOptics", "Tuning Step motor", "Aquisition", "Settings"}
  T2 = cluster{"Name":string, "Inicial":dbl, "Final":dbl}[]
  T3 = cluster{"WL Values":dbl[], "Spectrum Values":dbl[]}[]
  T4 = typedef "PowerMeterSteps.ctl" = enum16{"Initialize", "Graph", "Wait for Event", "Tuning", "Get Power", "MoveMotor", "corrects step"}
  T5 = typedef "OceanOptics.ctl" = enum16{"Initialize", "Graph", "Wait for Event", "Dark Spec", "Clear Dark Spec", "OceanOptics", "Create File", "Save"}
  T6 = enum16{"open", "replace", "create", "open or create", "replace or create", "replace or create with confirmation"}
  T7 = typedef "RL-Signal.ctl" = cluster{"Signal State":string, "Step":dbl, "Integration value":dbl, "Peak value":dbl, "Peak Wavelenght":dbl, "Spectrum values ":dbl[], "Error":errorcluster, "FWHM":dbl}
  T8 = cluster{"WL Values":dbl[], "Spectrum Values":dbl[]}
  T9 = cluster{"Wavelenght":dbl[], "Spectrum Values":dbl[]}
  T10 = typedef "NI_AALPro.lvlib/Integral Method.ctl" = i32
  T11 = cluster{"Wavelenght":dbl[], "Spectrum Values":dbl[]}[]
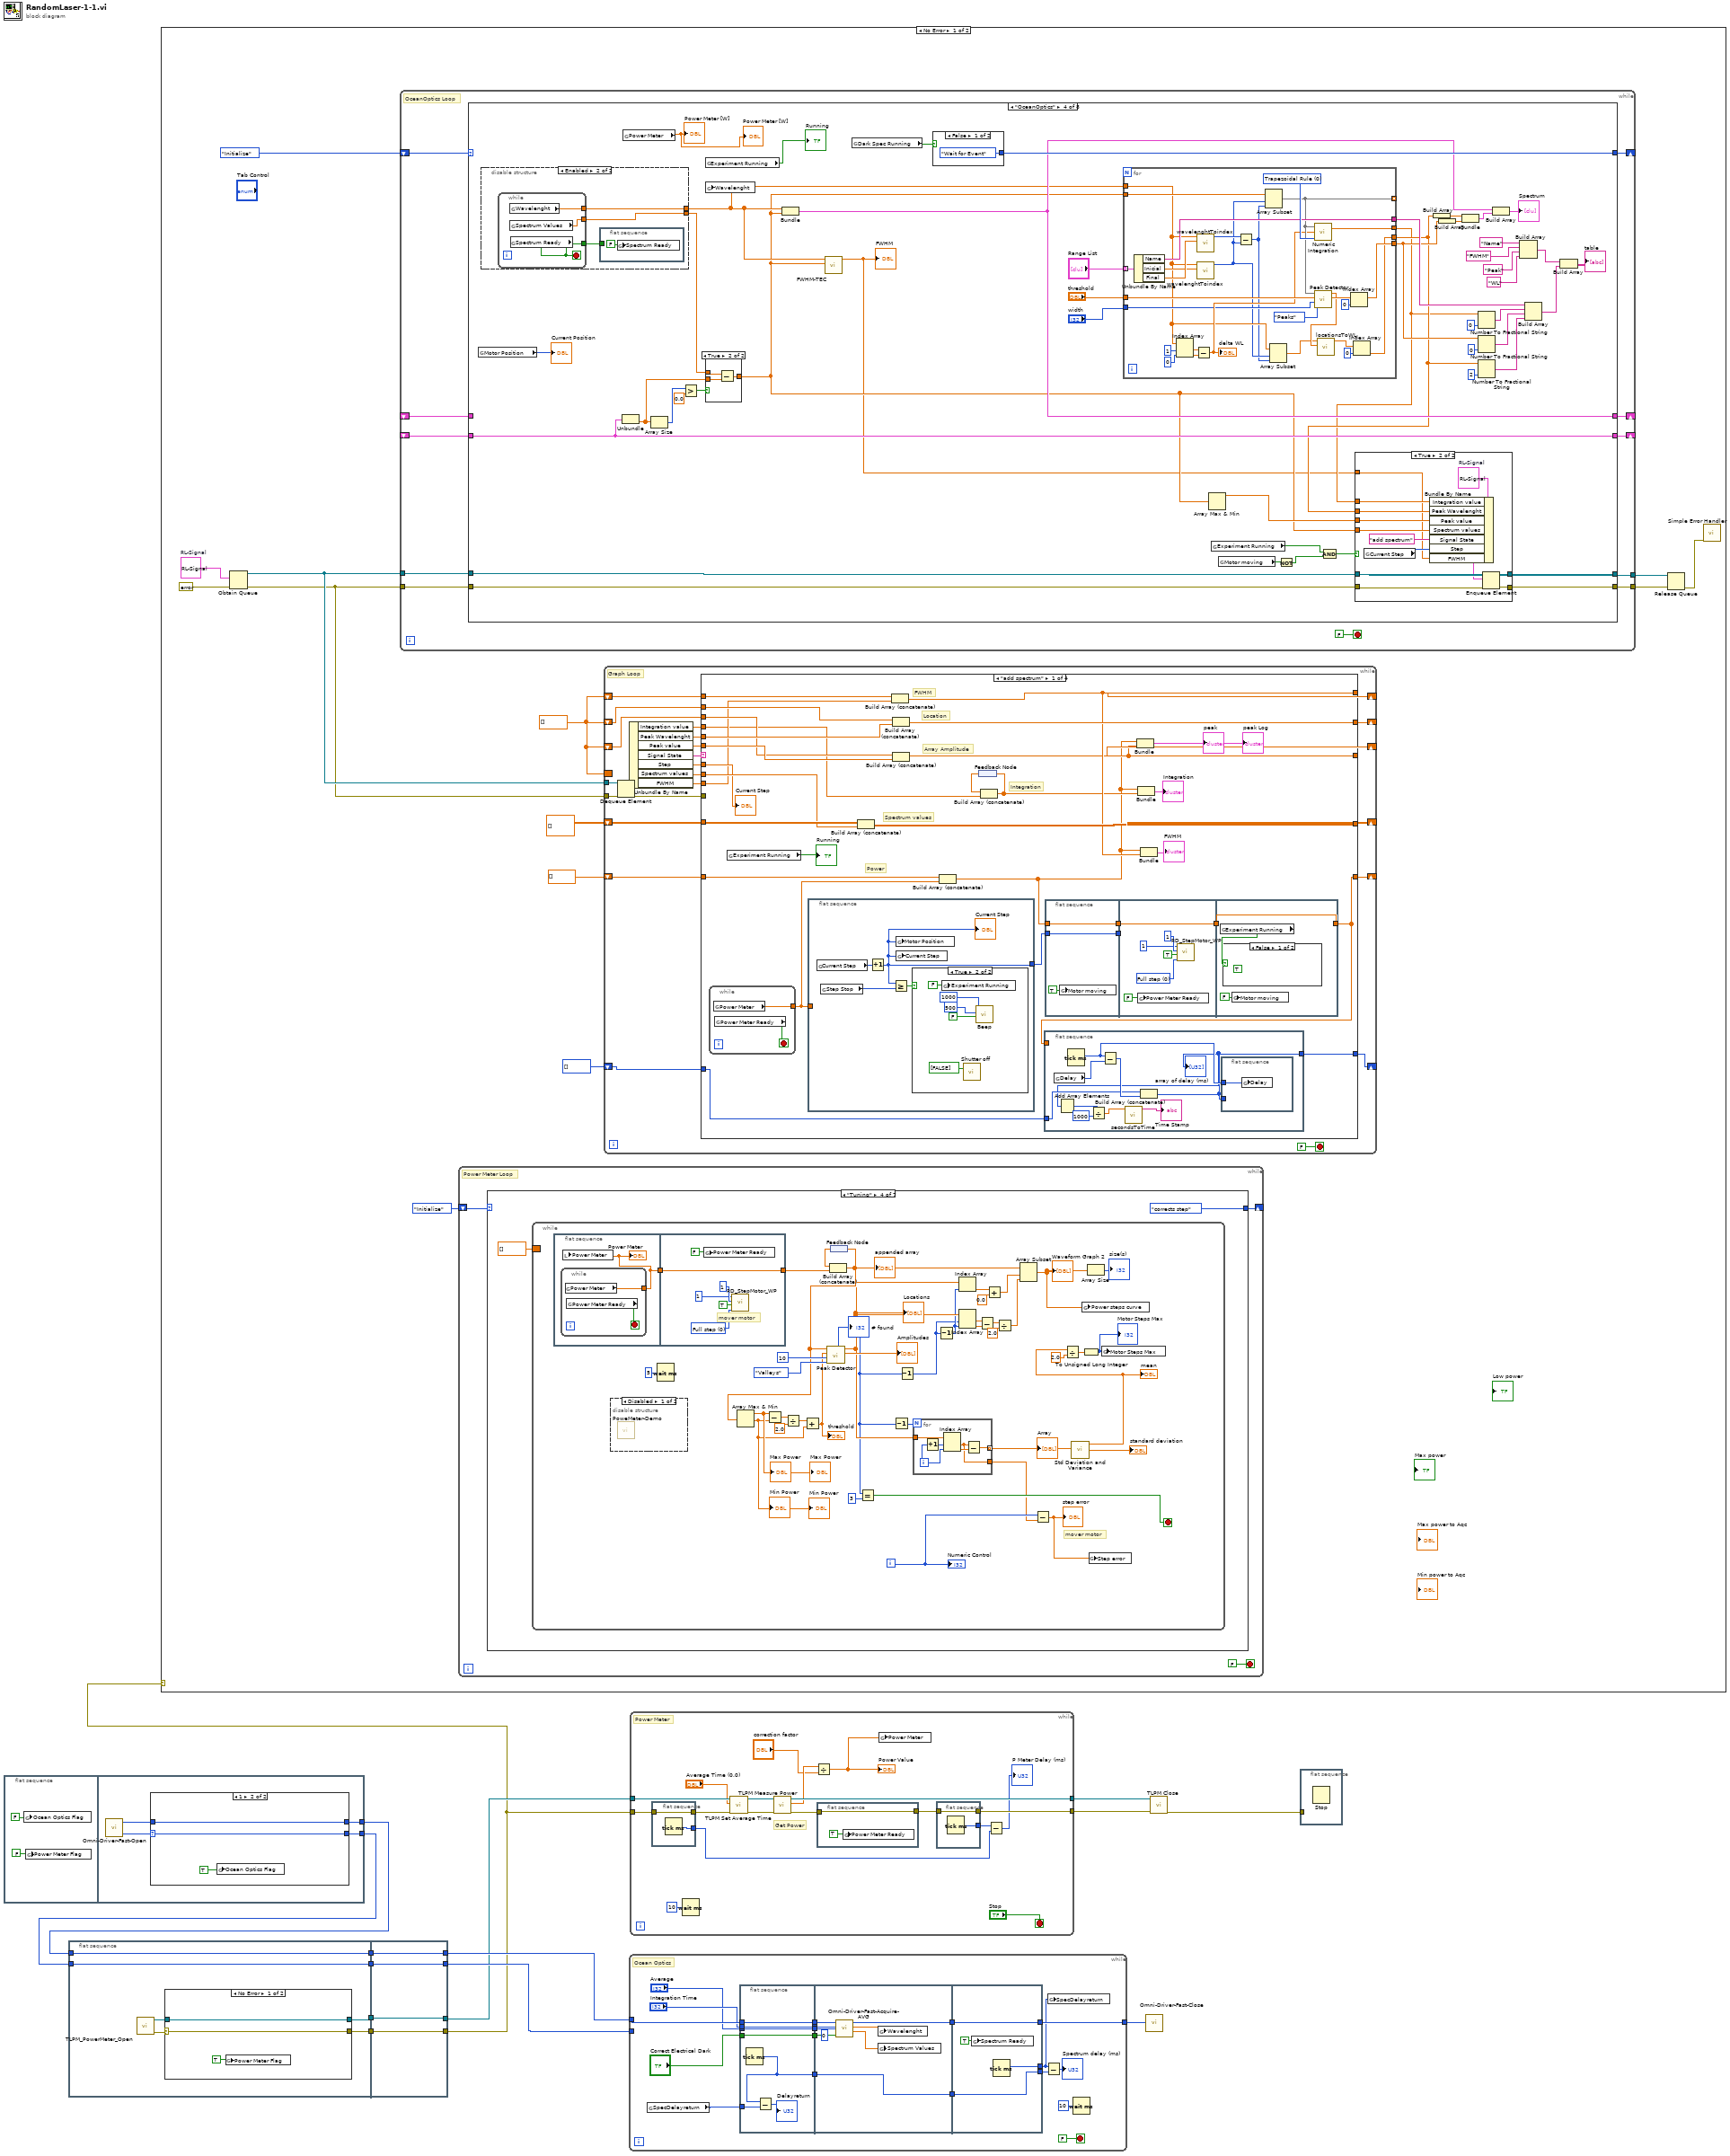
[diagram p0: block diagram]
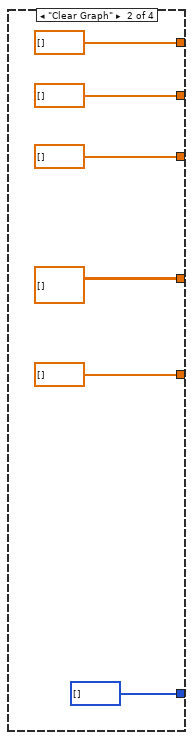
[diagram p4: hidden frame]
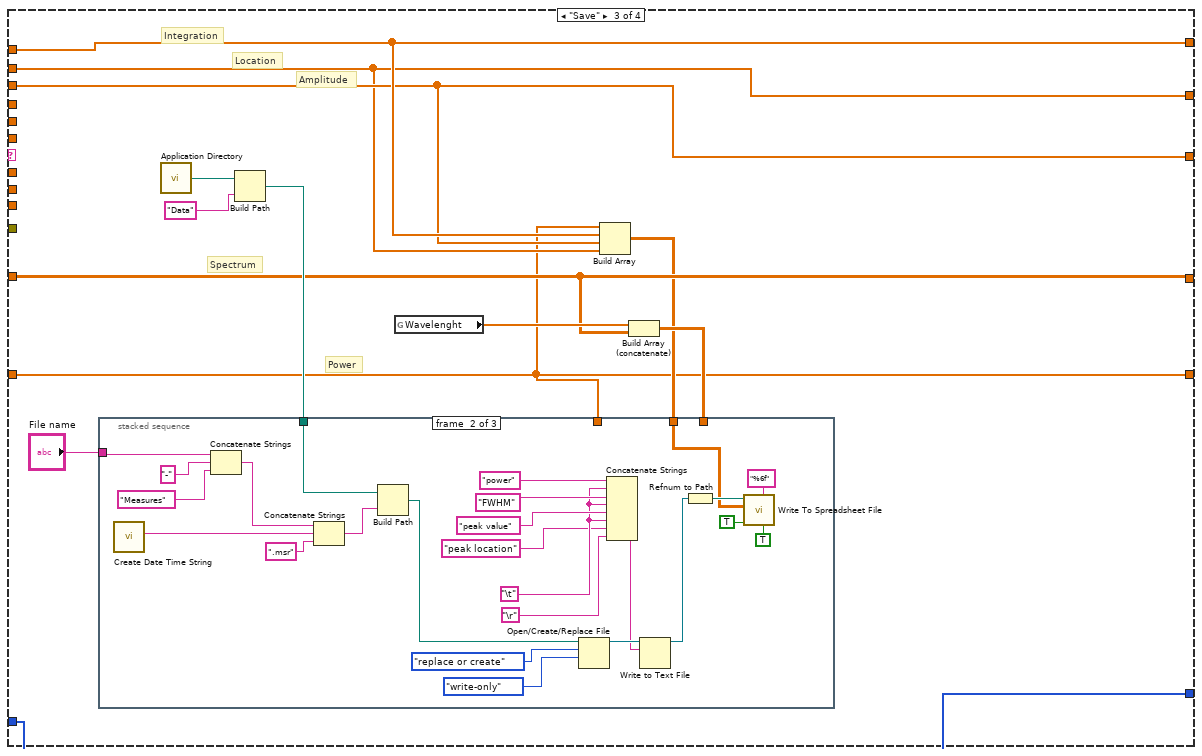
[diagram p5: hidden frame]
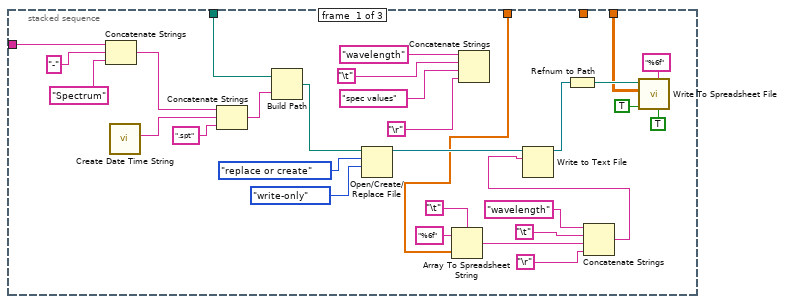
[diagram p6: hidden frame]
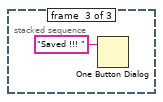
[diagram p7: hidden frame]
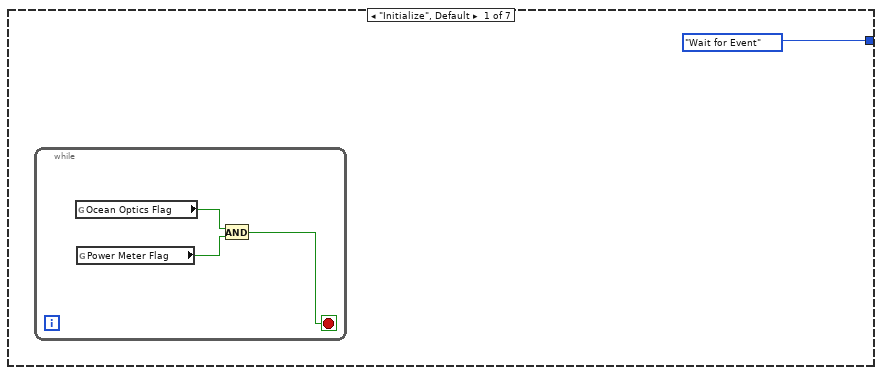
[diagram p9: hidden frame]
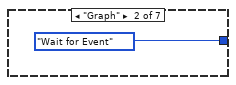
[diagram p10: hidden frame]
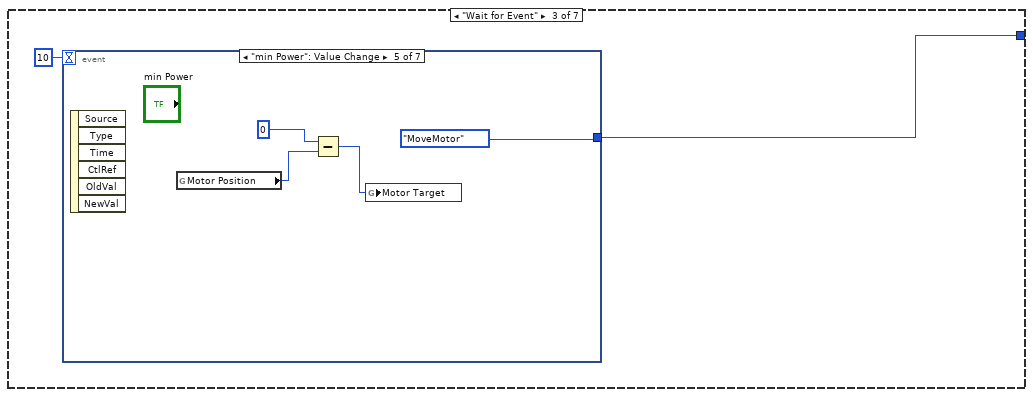
[diagram p11: hidden frame]
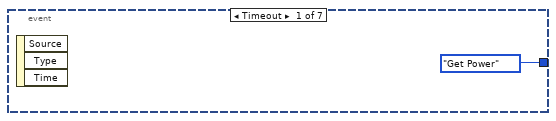
[diagram p12: hidden frame]
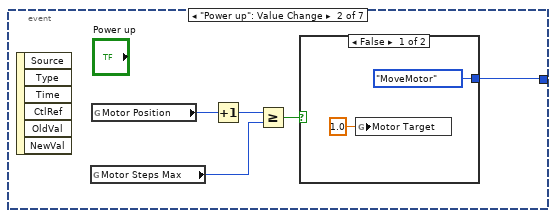
[diagram p13: hidden frame]
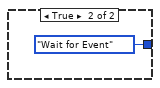
[diagram p14: hidden frame]
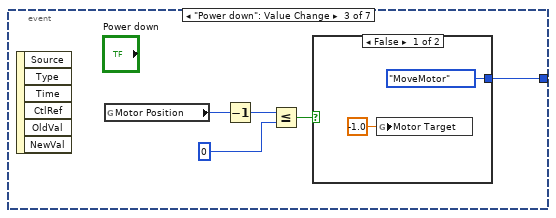
[diagram p15: hidden frame]
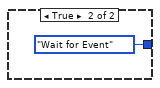
[diagram p16: hidden frame]
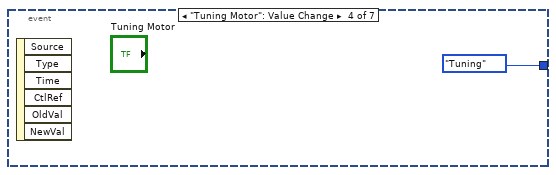
[diagram p17: hidden frame]
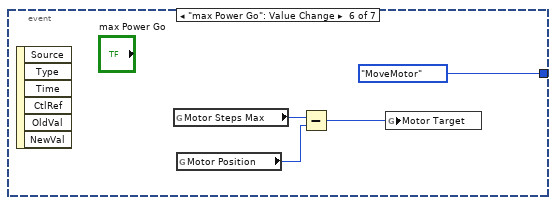
[diagram p18: hidden frame]
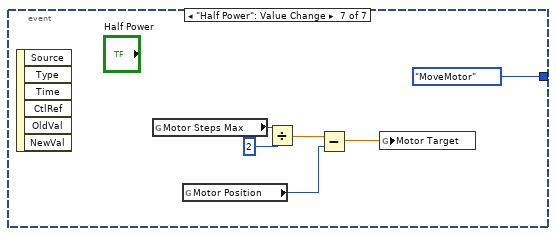
[diagram p19: hidden frame]
diagram:
  n1 = flat-sequence {
    tunnel: [w18] -> w8
    tunnel: [w17] -> w7
    frame #0 {
      n2 = global write "GlobalVariables.vi" "Ocean Optics Flag"(FALSE ("Ocean Optics")) -> ()
      n3 = global write "GlobalVariables.vi" "Power Meter Flag"(FALSE ("Ocean Optics")) -> ()
    }
    frame #1 {
      n4 = call "Omni-Driver-Fast-Open.vi"() -> ("Number of Spectrometers"=w20:i32, "Wrapper Out"=w19:u32)  [unwired: 4 in]
      n5 = case shown="1" w20 {
        selector: w20 -> [_ w23]
        tunnel: w19 -> [_ w24]
        tunnel: [_ w24] -> w18
        tunnel: [_ w23] -> w17
        frame 0, Default {
          n6 = flat-sequence {
            frame #0 {
              n7 = One Button Dialog(message="Ocean Optics not Connected") -> ()  [unwired: 1 in, 1 out]
            }
            frame #1 {
              n8 = Stop() -> ()  [unwired: 1 in]
            }
          }
        }
        frame 1 {
          n9 = global write "GlobalVariables.vi" "Ocean Optics Flag"(TRUE ("Ocean Optics")) -> ()
        }
      }
    }
  }
  n10 = flat-sequence {
    tunnel: [w28] -> w10
    tunnel: [w27] -> w9
    tunnel: w8 -> [w26]
    tunnel: w7 -> [w25]
    tunnel: [w26] -> w6
    tunnel: [w25] -> w3
    tunnel: w10 -> [w38]
    tunnel: [w38] -> w2
    tunnel: [w37] -> w1
    tunnel: w9 -> [w37]
    tunnel: [w36] -> w5
    tunnel: w6 -> [w36]
    tunnel: [w35] -> w4
    tunnel: w3 -> [w35]
    frame #0 {
      n11 = call "TLPM_PowerMeter_Open.vi"() -> ("error out"=w30:errorcluster, "instrument handle out"=w29:refnum<visa-resource-name>)  [unwired: 10 in]
      n12 = case shown="No Error" w30 {
        selector: w30 -> [w32 _]
        tunnel: w29 -> [w33 _]
        tunnel: [w33 _] -> w28
        tunnel: [w32 _] -> w27
        frame No Error {
          n13 = global write "GlobalVariables.vi" "Power Meter Flag"(TRUE ("Ocean Optics")) -> ()
        }
        frame Error {
          n14 = flat-sequence {
            frame #0 {
              n15 = One Button Dialog(message="Power Meter not Connected") -> ()  [unwired: 1 in, 1 out]
            }
            frame #1 {
              n16 = Stop() -> ()  [unwired: 1 in]
            }
          }
        }
      }
    }
    frame #1 {
    }
  }
  n17 = case shown="No Error" w1 {
    frame No Error {
      w39 = dbl[] []
      w48 = T7 {"Signal State"="", "Step"=0.0, "Integration value"=0.0, "Peak value"=0.0, "Peak Wavelenght"=0.0, "Spectrum values "=[], "Error"={"status"=FALSE, "code"=0, "source"=""}, "FWHM"=0.0}  # RL-Signal
      n18 = Obtain Queue(element data type=w48, error in (no error)=errorcluster {"status"=FALSE, "code"=0, "source"=""}) -> (queue out=w47:refnum<queue>, error out=w46:errorcluster)  [unwired: 3 in, 1 out]
      n19 = while {
        shift-right: [w353] -> _
        shift-left: OceanOptics."Initialize" -> [w350]
        shift-right: [w356] -> _
        shift-left: _ -> [w355]
        shift-right: [w352] -> _
        shift-left: _ -> [w351]
        tunnel: w46 -> [w349]
        tunnel: w47 -> [w348]
        tunnel: [w347] -> w42
        tunnel: [w346] -> w41
        stop <- FALSE stop-if-true
        # "OceanOptics Loop"
        n20 = case shown="\"OceanOptics\"" w350 {
          tunnel: [w360 w369 w377 w441 w514 w519 w522 w532] -> w356
          tunnel: w355 -> [_ w369 w377 _ w514 w519 w522 w532]
          tunnel: [OceanOptics."OceanOptics" OceanOptics."OceanOptics" w376 w444 OceanOptics."OceanOptics" OceanOptics."OceanOptics" OceanOptics."OceanOptics" OceanOptics."OceanOptics"] -> w353
          tunnel: [w360 w369 w374 w450 w513 w518 w521 w531] -> w352
          tunnel: w351 -> [_ _ w374 w450 w513 _ w521 w531]
          tunnel: w349 -> [w358 w365 w371 w438 w510 w515 w520 w535]
          tunnel: w348 -> [w359 w366 w373 w439 w511 w516 w528 w536]
          tunnel: [w359 w366 w372 w437 w511 w516 w525 w534] -> w347
          tunnel: [w358 w365 w370 w436 w510 w515 w524 w533] -> w346
          frame "Initialize", Default {
            w357 = 0 ("Motor Position")
            w360 = T8 {"WL Values"=[], "Spectrum Values"=[]}  # clear graph
            n21 = while {
              stop <- w362 stop-if-true
              n22 = global read "GlobalVariables.vi" "Ocean Optics Flag"() -> (w364:bool)
              n23 = global read "GlobalVariables.vi" "Power Meter Flag"() -> (w363:bool)
              n24 = And(x=w364, y=w363) -> (x .and. y?=w362:bool)
            }
            n25 = global write "GlobalVariables.vi" "Motor Position"(w357) -> ()
            n26 = global write "GlobalVariables.vi" "Current Step"(w357) -> ()
          }
          frame "Dark Spec" {
            n27 = global write "GlobalVariables.vi" "Dark Spec Running"(FALSE ("Dark Spec Running")) -> ()
          }
          frame "Wait for Event" {
            n28 = event shown="[2] \"Play Aquisition\": Value Change" {
              selector: _ -> [_ _ _ _ _]
              dyn-events: _ -> [_ _ _ _ _]
              timeout: 10 -> [_ _ _ _ _]
              tunnel: [OceanOptics."OceanOptics" OceanOptics."Clear Dark Spec" OceanOptics."OceanOptics" OceanOptics."Save" OceanOptics."Clear Dark Spec"] -> w376
              tunnel: w373 -> [w379 w382 w390 w398 w401]
              tunnel: w371 -> [w378 w381 w389 w397 w400]
              tunnel: [w379 w382 w388 w398 w401] -> w372
              tunnel: [w378 w381 w387 w397 w400] -> w370
              event Timeout {
                n29 = event-data() -> ()  [unwired: 1 in, 3 out]
              }
              event "Store Dark Spec": Value Change {
                n30 = event-data() -> ()  [unwired: 1 in, 3 out]
                n31 = global write "GlobalVariables.vi" "Dark Spec Running"(TRUE ("Dark Spec Running")) -> ()
              }
              event "Play Aquisition": Value Change {
                w392 = T7 {"Signal State"="", "Step"=0.0, "Integration value"=0.0, "Peak value"=0.0, "Peak Wavelenght"=0.0, "Spectrum values "=[], "Error"={"status"=FALSE, "code"=0, "source"=""}, "FWHM"=0.0}  # RL-Signal
                # "Mandar Clear Graph"
                n32 = event-data() -> ()  [unwired: 1 in, 3 out]
                n33 = Tick Count (ms)() -> (millisecond timer value=w386:u32)
                n34 = Bundle By Name(cluster=w392, "Signal State"="Clear Graph") -> (w391:T7)
                n35 = global write "GlobalVariables.vi" "Delay"(w386) -> ()
                n36 = Enqueue Element(queue=w390, element=w391, error in (no error)=w389) -> (queue out=w388:refnum<queue>, error out=w387:errorcluster)  [unwired: 1 in, 1 out]
                n37 = global write "GlobalVariables.vi" "Experiment Running"(TRUE ("Experiment Running")) -> ()
                n38 = global write "GlobalVariables.vi" "Step Stop"("Step Stop") -> ()
                n39 = call "Shutter on"("data"=bool[] [TRUE]) -> ()  [unwired: 17 in, 2 out]
              }
              event "Save Aquisition": Value Change {
                n40 = event-data() -> ()  [unwired: 1 in, 3 out]
              }
              event "Clear Dark Spec": Value Change {
                n41 = event-data() -> ()  [unwired: 1 in, 3 out]
              }
            }
          }
          frame "OceanOptics" {
            n42 = global read "GlobalVariables.vi" "Motor Position"() -> (→"Current Position":i32)
            n43 = disable-structure shown="Enabled" {
              disable-tunnel: [w481 w483] -> w446
              disable-tunnel: [w479 w484] -> w407
              frame Disabled {
                n44 = call "SpectrumOfLight.vi"("Select Light Source"="Select Light Source") -> ("Spectrum Values"=w481:dbl[], "WL Values"=w479:dbl[])  [unwired: 9 in]
              }
              frame Enabled {
                n45 = while {
                  tunnel: [w488] -> w484
                  tunnel: [w487] -> w483
                  tunnel: [w486] -> w482
                  stop <- w486 stop-if-true
                  n46 = global read "GlobalVariables.vi" "Wavelenght"() -> (w488:dbl[])
                  n47 = global read "GlobalVariables.vi" "Spectrum Values"() -> (w487:dbl[])
                  n48 = global read "GlobalVariables.vi" "Spectrum Ready"() -> (w486:bool)
                }
                n49 = flat-sequence {
                  tunnel: w482 -> [_]
                  frame #0 {
                    n50 = global write "GlobalVariables.vi" "Spectrum Ready"(FALSE ("Spectrum Ready")) -> ()
                  }
                }
              }
            }
            n51 = Unbundle(w450) -> ("Spectrum Values"=w445:dbl[])  [unwired: 1 out]
            n52 = global read "GlobalVariables.vi" "Power Meter"() -> (→"Power Meter [W]" →"Power Meter [W]":dbl)
            n53 = Array Size(array=w445) -> (size(s)=w447:i32)
            n54 = Greater?(x=w447, y=0.0) -> (0:w449:bool)
            n55 = global read "GlobalVariables.vi" "Experiment Running"() -> (→"Running":bool)
            n56 = case shown="True" w449 {
              tunnel: w446 -> [w506 w509]
              tunnel: w445 -> [_ w508]
              tunnel: [w506 w507] -> w405
              frame False {
              }
              frame True {
                n57 = Subtract(x=w509, y=w508) -> (x-y=w507:dbl[])
              }
            }
            n58 = global write "GlobalVariables.vi" "Wavelenght"(w407) -> ()
            n59 = Bundle("Wavelenght"=w407, "Spectrum Values"=w405) -> (w441:T9)  [unwired: 1 in]
            n60 = call "FWHM-TEC.vi"("Y values"=w405, "WL values"=w407) -> ("FWHM"=w403:dbl)  [unwired: 9 in]
            "FWHM" <- w403
            n61 = global read "GlobalVariables.vi" "Dark Spec Running"() -> (w443:bool)
            n62 = case shown="False" w443 {
              tunnel: [OceanOptics."Wait for Event" OceanOptics."Dark Spec"] -> w444
              frame False {
              }
              frame True {
              }
            }
            n63 = for {
              tunnel: w407 -> [w454]
              tunnel: w405 -> [w475]
              tunnel: "Range List" -> [w478] mode=indexing
              tunnel: [w470] -> _ mode=indexing
              tunnel: [w472] -> w404
              tunnel: [w471] -> w419
              tunnel: "threshold" -> [w469]
              tunnel: [w466] -> w416
              tunnel: "width" -> [w459]
              tunnel: [w455] -> w408
              w473 = T10 0 items=["Trapezoidal Rule", "Simpson's Rule", "Simpson's 3/8 Rule", "Bode Rule"] ("integration method")
              n64 = Unbundle By Name(w478) -> ("Name"=w471:string, "Inicial"=w476:dbl, "Final"=w477:dbl)
              n65 = Index Array(array=w454, index #1=1 ("index"), index #2=0 ("index")) -> (element #1=w461:dbl, element #2=w462:dbl)
              n66 = Subtract(x=w461, y=w462) -> (x-y=w460:dbl)
              "delta WL" <- w460
              n67 = call "wavelenghtToindex.vi"("WL in"=w477, "WL Values"=w454) -> ("index of WL"=w474:i32)  [unwired: 9 in]
              n68 = call "wavelenghtToindex.vi"("WL in"=w476, "WL Values"=w454) -> ("index of WL"=w452:i32)  [unwired: 9 in]
              n69 = Subtract(x=w474, y=w452) -> (x-y=w451:i32)
              n70 = Array Subset(array=w475, index=w452, length=w451) -> (w470:dbl[])
              n71 = Array Subset(array=w454, index=w452, length=w451) -> (w453:dbl[])
              n72 = call <vilib>:"Peak Detector.vi"("peaks/valleys"=enum32{"Peaks", "Valleys"}."Peaks", "width"=w459, "threshold"=w469, "X"=w470) -> ("Amplitudes"=w467:dbl[], "Locations"=w458:dbl[])  [unwired: 3 in, 3 out]
              n73 = call-poly <vilib>:"Numeric Integration.vi"("integration method"=w473, "dt"=w460, "Input Array"=w470) -> ("result"=w472:dbl)  [unwired: 1 out]
              n74 = call "locationsToWL.vi"("Locations index"=w458, "WL Values"=w453) -> ("Locations WL"=w456:dbl[])  [unwired: 9 in]
              n75 = Index Array(array=w467, index=0) -> (element=w466:dbl)
              n76 = Index Array(array=w456, index=0) -> (element=w455:dbl)
            }
            n77 = Array Max & Min(array=w405) -> (max value=w406:dbl)  [unwired: 3 out]
            n78 = global read "GlobalVariables.vi" "Experiment Running"() -> (w430:bool)
            n79 = global read "GlobalVariables.vi" "Motor moving"() -> (w432:bool)
            n80 = Not(x=w432) -> (.not. x?=w429:bool)
            n81 = And(x=w430, y=w429) -> (x .and. y?=w431:bool)
            n82 = case shown="True" w431 {
              tunnel: w439 -> [w490 w501]
              tunnel: w438 -> [w489 w500]
              tunnel: w405 -> [_ w498]
              tunnel: [w490 w497] -> w437
              tunnel: [w489 w496] -> w436
              tunnel: w404 -> [_ w494]
              tunnel: w408 -> [_ w493]
              tunnel: w406 -> [_ w492]
              tunnel: w403 -> [_ w491]
              frame False {
              }
              frame True {
                w503 = T7 {"Signal State"="", "Step"=0.0, "Integration value"=0.0, "Peak value"=0.0, "Peak Wavelenght"=0.0, "Spectrum values "=[], "Error"={"status"=FALSE, "code"=0, "source"=""}, "FWHM"=0.0}  # RL-Signal
                n83 = global read "GlobalVariables.vi" "Current Step"() -> (w495:i32)
                n84 = Bundle By Name(cluster=w503, "Integration value"=w494, "Peak Wavelenght"=w493, "Peak value"=w492, "Spectrum values"=w498, "Signal State"="add spectrum", "Step"=w495, "FWHM"=w491) -> (w499:T7)
                n85 = Enqueue Element(queue=w501, element=w499, error in (no error)=w500) -> (queue out=w497:refnum<queue>, error out=w496:errorcluster)  [unwired: 1 in, 1 out]
              }
            }
            n86 = Build Array(w408) -> (w418:dbl[])
            n87 = Build Array(w416) -> (w417:dbl[])
            n88 = Bundle(w418, w417) -> (w442:cluster{dbl[], dbl[]})  [unwired: 1 in]
            n89 = Number To Fractional String(number=w404, precision (6)=i16 0) -> (F-format string=w413:string)  [unwired: 2 in]
            n90 = Number To Fractional String(number=w416, precision (6)=i16 0) -> (F-format string=w412:string)  [unwired: 2 in]
            n91 = Number To Fractional String(number=w408, precision (6)=i16 2) -> (F-format string=w409:string)  [unwired: 2 in]
            n92 = Build Array(w441, w442) -> (→"Spectrum":T11)
            n93 = Build Array("Name", "FWHM", "Peak", "WL") -> (w425:string[])
            n94 = Build Array(w419, w413, w412, w409) -> (w422:string[])
            n95 = Build Array(w425, w422) -> (→"table":string[][])
          }
          frame "Graph" {
          }
          frame "Clear Dark Spec" {
            w518 = T8 {"WL Values"=[], "Spectrum Values"=[]}  # clear graph
          }
          frame "Create File" {
            w527 = T7 {"Signal State"="", "Step"=0.0, "Integration value"=0.0, "Peak value"=0.0, "Peak Wavelenght"=0.0, "Spectrum values "=[], "Error"={"status"=FALSE, "code"=0, "source"=""}, "FWHM"=0.0}  # RL-Signal
            n96 = Bundle By Name(cluster=w527, "Signal State"="Create File") -> (w526:T7)
            n97 = Enqueue Element(queue=w528, element=w526, error in (no error)=w520) -> (queue out=w525:refnum<queue>, error out=w524:errorcluster)  [unwired: 1 in, 1 out]
          }
          frame "Save" {
            w538 = T7 {"Signal State"="", "Step"=0.0, "Integration value"=0.0, "Peak value"=0.0, "Peak Wavelenght"=0.0, "Spectrum values "=[], "Error"={"status"=FALSE, "code"=0, "source"=""}, "FWHM"=0.0}  # RL-Signal
            n98 = Bundle By Name(cluster=w538, "Signal State"="Save") -> (w537:T7)
            n99 = Enqueue Element(queue=w536, element=w537, error in (no error)=w535) -> (queue out=w534:refnum<queue>, error out=w533:errorcluster)  [unwired: 1 in, 1 out]
          }
        }
      }
      n100 = while {
        shift-right: [w220] -> _
        shift-left: PowerMeterSteps."Initialize" ("Enum") -> [w221]
        stop <- FALSE stop-if-true
        # "Power Meter Loop"
        n101 = case shown="\"Tuning\"" w221 {
          tunnel: [PowerMeterSteps."Wait for Event" ("Enum") PowerMeterSteps."Wait for Event" ("Enum") w229 PowerMeterSteps."corrects step" ("Enum") PowerMeterSteps."Wait for Event" ("Enum") PowerMeterSteps."Wait for Event" ("Enum") PowerMeterSteps."Wait for Event" ("Enum")] -> w220
          frame "Initialize", Default {
            n102 = while {
              stop <- w224 stop-if-true
              n103 = global read "GlobalVariables.vi" "Ocean Optics Flag"() -> (w226:bool)
              n104 = global read "GlobalVariables.vi" "Power Meter Flag"() -> (w225:bool)
              n105 = And(x=w226, y=w225) -> (x .and. y?=w224:bool)
            }
          }
          frame "Graph" {
          }
          frame "Wait for Event" {
            n106 = event shown="[4] \"min Power\": Value Change" {
              selector: _ -> [_ _ _ _ _ _ _]
              dyn-events: _ -> [_ _ _ _ _ _ _]
              timeout: 10 -> [_ _ _ _ _ _ _]
              tunnel: [PowerMeterSteps."Get Power" ("Enum") w232 w239 PowerMeterSteps."Tuning" ("Enum") PowerMeterSteps."MoveMotor" ("Enum") PowerMeterSteps."MoveMotor" ("Enum") PowerMeterSteps."MoveMotor" ("Enum")] -> w229
              event Timeout {
                n107 = event-data() -> ()  [unwired: 1 in, 3 out]
              }
              event "Power up": Value Change {
                n108 = event-data() -> ()  [unwired: 1 in, 6 out]
                n109 = global read "GlobalVariables.vi" "Motor Steps Max"() -> (w234:i32)
                n110 = global read "GlobalVariables.vi" "Motor Position"() -> (w235:i32)
                n111 = Increment(x=w235) -> (x+1=w231:i32)
                n112 = Greater Or Equal?(x=w231, y=w234) -> (x >= y?=w233:bool)
                n113 = case shown="False" w233 {
                  tunnel: [PowerMeterSteps."MoveMotor" ("Enum") PowerMeterSteps."Wait for Event" ("Enum")] -> w232
                  frame False {
                    n114 = global write "GlobalVariables.vi" "Motor Target"(1.0 ("Motor Target")) -> ()
                  }
                  frame True {
                  }
                }
              }
              event "Power down": Value Change {
                n115 = event-data() -> ()  [unwired: 1 in, 6 out]
                n116 = global read "GlobalVariables.vi" "Motor Position"() -> (w241:i32)
                n117 = Decrement(x=w241) -> (x-1=w243:i32)
                n118 = Less Or Equal?(x=w243, y=0) -> (x <= y?=w242:bool)
                n119 = case shown="False" w242 {
                  tunnel: [PowerMeterSteps."MoveMotor" ("Enum") PowerMeterSteps."Wait for Event" ("Enum")] -> w239
                  frame False {
                    n120 = global write "GlobalVariables.vi" "Motor Target"(-1.0 ("Motor Target")) -> ()
                  }
                  frame True {
                  }
                }
              }
              event "Tuning Motor": Value Change {
                n121 = event-data() -> ()  [unwired: 1 in, 6 out]
              }
              event "min Power": Value Change {
                n122 = event-data() -> ()  [unwired: 1 in, 6 out]
                n123 = global read "GlobalVariables.vi" "Motor Position"() -> (w249:i32)
                n124 = Subtract(x=0, y=w249) -> (x-y=w248:i32)
                n125 = global write "GlobalVariables.vi" "Motor Target"(w248) -> ()
              }
              event "max Power Go": Value Change {
                n126 = event-data() -> ()  [unwired: 1 in, 6 out]
                n127 = global read "GlobalVariables.vi" "Motor Steps Max"() -> (w254:i32)
                n128 = global read "GlobalVariables.vi" "Motor Position"() -> (w253:i32)
                n129 = Subtract(x=w254, y=w253) -> (x-y=w252:i32)
                n130 = global write "GlobalVariables.vi" "Motor Target"(w252) -> ()
              }
              event "Half Power": Value Change {
                n131 = event-data() -> ()  [unwired: 1 in, 6 out]
                n132 = global read "GlobalVariables.vi" "Motor Steps Max"() -> (w260:i32)
                n133 = global read "GlobalVariables.vi" "Motor Position"() -> (w257:i32)
                n134 = Divide(x=w260, y=2) -> (x/y=w258:dbl)
                n135 = Subtract(x=w258, y=w257) -> (x-y=w256:dbl)
                n136 = global write "GlobalVariables.vi" "Motor Target"(w256) -> ()
              }
            }
          }
          frame "Tuning" {
            n137 = while {
              border: dbl[] [] -> [_]
              i -> [w289]
              stop <- w292 stop-if-true
              # "mover motor"
              n138 = flat-sequence {
                tunnel: [w304] -> w283
                tunnel: [w312] -> w284
                tunnel: w283 -> [w312]
                frame #0 {
                  n139 = while {
                    tunnel: [w305] -> w304
                    stop <- w306 stop-if-true
                    n140 = global read "GlobalVariables.vi" "Power Meter"() -> (w305:dbl)
                    n141 = global read "GlobalVariables.vi" "Power Meter Ready"() -> (w306:bool)
                  }
                  "Power Meter" <- w304
                  n142 = local write "Power Meter"(w304) -> ()
                }
                frame #1 {
                  w309 = u16 0 items=["Full step", "Half step", "1/4 step", "1/8 step", "1/16 step", "1/32 step"] ("Step resolution")
                  # "mover motor"
                  n143 = global write "GlobalVariables.vi" "Power Meter Ready"(FALSE ("Power Meter Ready")) -> ()
                  n144 = call "RD_StepMotor_WP.vi"("Step resolution"=w309, "Direction"=TRUE, "Time between steps (ms)"=1, "Steps"=i64 1) -> ()  [unwired: 8 in]
                }
              }
              n145 = disable-structure shown="Disabled" {
                frame Disabled {
                  n146 = call "PoweMeter-Demo.vi"() -> ()  [unwired: 10 in, 2 out]
                }
                frame Enabled {
                }
              }
              n147 = Wait (ms)(milliseconds to wait=u32 5) -> ()  [unwired: 1 out]
              n148 = feedback #1() -> (w303:dbl[])
              n149 = Build Array (concatenate)(w303, w284) -> (w279:dbl[])
              "appended array" <- w279
              n150 = Array Max & Min(array=w279) -> (max value=w281:dbl, min value=w280:dbl)  [unwired: 2 out]
              "Max Power" <- w281
              "Min Power" <- w280
              "Min Power" <- w280
              "Max Power" <- w281
              n151 = Subtract(x=w281, y=w280) -> (x-y=w296:dbl)
              n152 = Divide(x=w296, y=2.0) -> (x/y=w294:dbl)
              n153 = Add(x=w294, y=w280) -> (x+y=w297:dbl)
              "threshold" <- w297
              n154 = call <vilib>:"Peak Detector.vi"("peaks/valleys"=enum32{"Peaks", "Valleys"}."Valleys", "width"=10 ("width 2"), "threshold"=w297, "X"=w279) -> ("Amplitudes"=→"Amplitudes":dbl[], "Locations"=w278:dbl[], "# found"=w268:i32)  [unwired: 3 in, 2 out]
              "# found" <- w268
              "Locations" <- w278
              n155 = feedback-in #1(w279) -> ()
              n156 = Equal?(x=w268, y=3) -> (x = y?=w292:bool)
              n157 = Decrement(x=w268) -> (x-1=w300:i32)
              n158 = Decrement(x=w268) -> (x-1=w266:i32)
              n159 = for {
                N: w300 -> [_]
                tunnel: w278 -> [w318]
                tunnel: [w314] -> w299 mode=indexing
                tunnel: [w313] -> w288
                i -> [w316]
                n160 = Increment(x=w316) -> (x+1=w317:i32)
                n161 = Index Array(array=w318, index #1=w317, index #2=w316) -> (element #1=w313:dbl, element #2=w315:dbl)
                n162 = Subtract(x=w313, y=w315) -> (x-y=w314:dbl)
              }
              "Array" <- w299
              n163 = Decrement(x=w266) -> (x-1=w267:i32)
              n164 = Index Array(array=w278, index=w267) -> (element=w275:dbl)
              n165 = Index Array(array=w278, index #1=w266, index #2=w267) -> (element #1=w276:dbl, element #2=w277:dbl)
              n166 = Subtract(x=w276, y=w277) -> (x-y=w272:dbl)
              n167 = Add(x=w275, y=0.0) -> (x+y=w274:dbl)
              n168 = Divide(x=w272, y=2.0) -> (x/y=w273:dbl)
              n169 = Array Subset(array=w279, index=w274, length=w273) -> (w265:dbl[])
              "Waveform Graph 2" <- w265
              n170 = Subtract(x=w289, y=w288) -> (x-y=w282:dbl)
              "step error" <- w282
              n171 = call <vilib>:"Std Deviation and Variance.vi"("X"=w299) -> ("mean"=w286:dbl, "standard deviation"=→"standard deviation":dbl)  [unwired: 1 in, 1 out]
              "mean" <- w286
              n172 = Divide(x=w286, y=2.0) -> (x/y=w285:dbl)
              n173 = global write "GlobalVariables.vi" "Power steps curve"(w265) -> ()
              n174 = To Unsigned Long Integer(number=w285) -> (unsigned 32bit integer=w264:u32)
              "Motor Steps Max" <- w264
              n175 = Array Size(array=w265) -> (size(s)=→"size(s)":i32)
              n176 = global write "GlobalVariables.vi" "Step error"(w282) -> ()
              n177 = global write "GlobalVariables.vi" "Motor Steps Max"(w264) -> ()
              "Numeric Control" <- w289
            }
          }
          frame "Get Power" {
            n178 = disable-structure shown="Disabled" {
              frame Disabled {
                n179 = call "PoweMeter-Demo.vi"("reset"=TRUE) -> ()  [unwired: 9 in, 2 out]
              }
              frame Enabled {
              }
            }
            n180 = flat-sequence {
              frame #0 {
                n181 = while {
                  stop <- w320 stop-if-true
                  n182 = global read "GlobalVariables.vi" "Power Meter"() -> (→"Power Meter":dbl)
                  n183 = global read "GlobalVariables.vi" "Power Meter Ready"() -> (w320:bool)
                }
              }
              frame #1 {
                n184 = global write "GlobalVariables.vi" "Power Meter Ready"(FALSE ("Power Meter Ready")) -> ()
              }
            }
          }
          frame "MoveMotor" {
            n185 = global read "GlobalVariables.vi" "Motor Position"() -> (w330:i32)
            n186 = global read "GlobalVariables.vi" "Motor Target"() -> (w329:dbl)
            n187 = global read "GlobalVariables.vi" "Motor Steps Max"() -> (w328:i32)
            n188 = Add(x=w330, y=w329) -> (x+y=w326:dbl)
            n189 = Increment(x=w328) -> (x+1=w324:i32)
            n190 = Greater?(x=w329, y=0.0) -> (0:w332:bool)
            n191 = Absolute Value(x=w329) -> (abs(x)=w333:dbl)
            n192 = In Range and Coerce(upper limit=w324, x=w326, lower limit=0) -> (In Range?=w325:bool)  [unwired: 1 out]
            n193 = case shown="True" w325 {
              tunnel: w333 -> [_ w339]
              tunnel: w332 -> [_ w338]
              tunnel: w326 -> [_ w335]
              frame False {
              }
              frame True {
                w337 = u16 0 items=["Full step", "Half step", "1/4 step", "1/8 step", "1/16 step", "1/32 step"] ("Step resolution")
                # "Atualiza posição Motor"
                # "LOOP de Mover o Motor"
                n194 = call "RD_StepMotor_WP.vi"("Step resolution"=w337, "Direction"=w338, "Time between steps (ms)"=10, "Steps"=w339) -> ()  [unwired: 8 in]
                n195 = global write "GlobalVariables.vi" "Motor Position"(w335) -> ()
                n196 = global write "GlobalVariables.vi" "Current Step"(w335) -> ()
                "Motor Target" <- w335
              }
            }
          }
          frame "corrects step" {
            w343 = u16 0 items=["Full step", "Half step", "1/4 step", "1/8 step", "1/16 step", "1/32 step"] ("Step resolution")
            n197 = global read "GlobalVariables.vi" "Step error"() -> (w342:i32)
            n198 = global write "GlobalVariables.vi" "Motor Position"(0 ("Current Step")) -> ()
            n199 = call "RD_StepMotor_WP.vi"("Step resolution"=w343, "Direction"=FALSE, "Time between steps (ms)"=10, "Steps"=w342) -> ()  [unwired: 8 in]
          }
        }
      }
      n200 = while {
        tunnel: w47 -> [w74]
        tunnel: w46 -> [w73]
        shift-right: [w66] -> _
        shift-left: dbl[][] [] -> [w71]
        shift-right: [w61] -> _
        shift-left: w39 -> [w62]
        shift-right: [w59] -> _
        shift-left: w39 -> [w60]
        shift-right: [w57] -> _
        shift-left: w39 -> [w58]
        shift-right: [w55] -> _
        shift-left: dbl[] [] -> [w56]
        shift-right: [w53] -> _
        shift-left: u32[] [] -> [w54]
        border: w39 -> [_]
        stop <- FALSE stop-if-true
        # "Graph Loop"
        n201 = Dequeue Element(queue=w74, error in (no error)=w73) -> (element=w70:T7, error out=w72:errorcluster)  [unwired: 1 in, 2 out]
        n202 = Unbundle By Name(w70) -> ("Integration value"=w65:dbl, "Peak Wavelenght"=w64:dbl, "Peak value"=w63:dbl, "Signal State"=w69:string, "Step"=w67:dbl, "Spectrum values"=w68:dbl[], "FWHM"=w52:dbl)
        n203 = case shown="\"add spectrum\"" w69 {
          tunnel: w72 -> [_ _ _ _]
          tunnel: w71 -> [w105 _ w152 w219]
          tunnel: w68 -> [w91 _ _ _]
          tunnel: w67 -> [w88 _ _ _]
          tunnel: [w104 dbl[][] [] w152 w219] -> w66
          tunnel: w65 -> [w80 _ _ _]
          tunnel: w64 -> [w103 _ _ _]
          tunnel: w63 -> [w102 _ _ _]
          tunnel: w62 -> [w101 _ w150 w218]
          tunnel: [w90 dbl[] [] w150 w218] -> w61
          tunnel: w60 -> [w100 _ w148 w217]
          tunnel: [w99 dbl[] [] w148 w217] -> w59
          tunnel: w58 -> [w98 _ w149 w216]
          tunnel: [w77 dbl[] [] w149 w216] -> w57
          tunnel: w56 -> [w97 _ w146 w215]
          tunnel: [w86 dbl[] [] w146 w215] -> w55
          tunnel: w54 -> [w85 _ w145 w214]
          tunnel: [w84 u32[] [] w145 w214] -> w53
          tunnel: w52 -> [w82 _ _ _]
          frame "add spectrum" {
            # "Integration"
            # "Spectrum values"
            # "Power"
            # "Array Amplitude"
            # "Location"
            # "FWHM"
            n204 = while {
              tunnel: [w125] -> w96
              stop <- w126 stop-if-true
              n205 = global read "GlobalVariables.vi" "Power Meter"() -> (w125:dbl)
              n206 = global read "GlobalVariables.vi" "Power Meter Ready"() -> (w126:bool)
            }
            n207 = global read "GlobalVariables.vi" "Experiment Running"() -> (→"Running":bool)
            n208 = flat-sequence {
              tunnel: w96 -> [_]
              tunnel: [w116] -> w95
              frame #0 {
                n209 = global read "GlobalVariables.vi" "Current Step"() -> (w119:i32)
                n210 = global read "GlobalVariables.vi" "Step Stop"() -> (w118:i32)
                n211 = Increment(x=w119) -> (x+1=w116:i32)
                "Current Step" <- w116
                n212 = Greater Or Equal?(x=w116, y=w118) -> (x >= y?=w117:bool)
                n213 = global write "GlobalVariables.vi" "Motor Position"(w116) -> ()
                n214 = global write "GlobalVariables.vi" "Current Step"(w116) -> ()
                n215 = case shown="True" w117 {
                  frame False {
                  }
                  frame True {
                    n216 = global write "GlobalVariables.vi" "Experiment Running"(FALSE ("Experiment Running")) -> ()
                    n217 = call "Shutter off"("data"=bool[] [FALSE]) -> ()  [unwired: 17 in, 2 out]
                    n218 = call <vilib>:"Beep.vi"("use system alert? (T)"=FALSE, "duration (msec)"=u32 500, "frequency (Hz)"=u32 1000) -> ()  [unwired: 9 in]
                  }
                }
              }
            }
            n219 = Build Array (concatenate)(w105, w91) -> (w104:dbl[][])
            n220 = Build Array (concatenate)(w101, w82) -> (w90:dbl[])
            n221 = Build Array (concatenate)(w100, w103) -> (w99:dbl[])
            n222 = Build Array (concatenate)(w98, w102) -> (w77:dbl[])
            n223 = Build Array (concatenate)(w97, w96) -> (w78:dbl[])
            n224 = feedback #2() -> (w81:dbl[])
            n225 = Build Array (concatenate)(w81, w80) -> (w79:dbl[])
            n226 = feedback-in #2(w79) -> ()
            n227 = flat-sequence {
              tunnel: w86 -> [_]
              tunnel: w85 -> [w107]
              tunnel: [w106] -> w84
              frame #0 {
                n228 = global read "GlobalVariables.vi" "Delay"() -> (w114:u32)
                n229 = Tick Count (ms)() -> (millisecond timer value=w112:u32)
                n230 = Subtract(x=w112, y=w114) -> (x-y=w113:u32)
                n231 = Build Array (concatenate)(w107, w113) -> (w106:u32[])
                "array of delay (ms)" <- w106
                n232 = Add Array Elements(numeric array=w106) -> (sum=w111:u32)
                n233 = Divide(x=w111, y=u32 1000) -> (x/y=w109:dbl)
                n234 = call "secondsToTime.vi"("Time input (s)"=w109) -> ("Time Stamp"=→"Time Stamp":string)  [unwired: 10 in]
                n235 = flat-sequence {
                  tunnel: w106 -> [_]
                  tunnel: w112 -> [w115]
                  frame #0 {
                    n236 = global write "GlobalVariables.vi" "Delay"(w115) -> ()
                  }
                }
              }
            }
            n237 = flat-sequence {
              tunnel: w95 -> [w128]
              tunnel: w78 -> [w129]
              tunnel: [w129] -> w94
              tunnel: [w128] -> w93
              tunnel: w94 -> [w135]
              tunnel: w93 -> [_]
              tunnel: [w135] -> w92
              tunnel: [w138] -> w86
              tunnel: w92 -> [w138]
              frame #0 {
                n238 = global write "GlobalVariables.vi" "Motor moving"(TRUE ("Motor moving")) -> ()
              }
              frame #1 {
                w132 = u16 0 items=["Full step", "Half step", "1/4 step", "1/8 step", "1/16 step", "1/32 step"] ("Step resolution")
                n239 = global write "GlobalVariables.vi" "Power Meter Ready"(FALSE ("Power Meter Ready")) -> ()
                n240 = call "RD_StepMotor_WP.vi"("Step resolution"=w132, "Direction"=TRUE, "Time between steps (ms)"=1, "Steps"=i64 1) -> ()  [unwired: 8 in]
              }
              frame #2 {
                n241 = global read "GlobalVariables.vi" "Experiment Running"() -> (w136:bool)
                n242 = case shown="False" w136 {
                  frame False {
                    (unwired) TRUE ("min Power")
                  }
                  frame True {
                  }
                }
                n243 = global write "GlobalVariables.vi" "Motor moving"(FALSE ("Motor moving")) -> ()
              }
            }
            n244 = Bundle(w78, w77) -> (→"peak Log" →"peak":cluster{dbl[], dbl[]})  [unwired: 1 in]
            n245 = Bundle(w78, w79) -> (→"Integration":cluster{dbl[], dbl[]})  [unwired: 1 in]
            n246 = Bundle(w78, w90) -> (→"FWHM":cluster{dbl[], dbl[]})  [unwired: 1 in]
            "Current Step" <- w88
          }
          frame "Clear Graph" {
          }
          frame "Save" {
            # "Spectrum"
            # "Power"
            # "Amplitude"
            # "Location"
            # "Integration"
            n247 = call <vilib>:"Application Directory.vi"() -> ("Application Directory"=w156:path)
            n248 = Build Path(base path=w156, name or relative path="Data" ("prompt (Create Folder)")) -> (appended path=w155:path)
            n249 = global read "GlobalVariables.vi" "Wavelenght"() -> (w154:dbl[])
            n250 = Build Array(w146, w150, w149, w148) -> (w151:dbl[][])
            n251 = Build Array (concatenate)(w154, w152) -> (w153:dbl[][])
            n252 = stacked-sequence {
              tunnel: w155 -> [w181 w202 _]
              tunnel: w153 -> [w177 _ _]
              tunnel: w151 -> [_ w201 _]
              tunnel: "File name" -> [w176 w199 _]
              tunnel: w146 -> [w163 _ _]
              frame #0 {
                n253 = Concatenate Strings(w176, "-", "Spectrum" ("string")) -> (w173:string)
                n254 = call "Create Date Time String.vi"() -> ("Date/Time String"=w180:string)  [unwired: 10 in, 1 out]
                n255 = Concatenate Strings(w173, w180, ".spt" ("string")) -> (w178:string)
                n256 = Build Path(base path=w181, name or relative path=w178) -> (appended path=w185:path)
                n257 = Open/Create/Replace File(file path (use dialog)=w185, operation (0:open)=T6."replace or create", access (0:read/write)=enum16{"read/write", "read-only", "write-only"}."write-only") -> (refnum out=w172:refnum<file>)  [unwired: 3 in, 2 out]
                n258 = Array To Spreadsheet String(delimiter (Tab)="\t", array=w163, 3:"%6f" ("format string")) -> (spreadsheet string=w162:string)
                n259 = Concatenate Strings("wavelength" ("string"), "\t", "spec values" ("string"), "\r") -> ()  [unwired: 1 out]
                n260 = Concatenate Strings("wavelength" ("string"), "\t", w162, "\r") -> (w161:string)
                n261 = Write to Text File(file (use dialog)=w172, text=w161) -> (refnum out=w171:refnum<file>)  [unwired: 2 in, 2 out]
                n262 = Refnum to Path(1:w171) -> (0:w187:path)
                n263 = call-poly <vilib>:"Write To Spreadsheet File.vi"("transpose? (no:F)"=TRUE, "format (%.3f)"="%6f" ("format string"), "append to file? (new file:F)"=TRUE, "2D data"=w177, "file path (dialog if empty)"=w187) -> ()  [unwired: 3 in, 1 out]
              }
              frame #1 {
                w192 = "\t"
                n264 = call "Create Date Time String.vi"() -> ("Date/Time String"=w205:string)  [unwired: 10 in, 1 out]
                n265 = Concatenate Strings(w199, "-", "Measures" ("string")) -> (w197:string)
                n266 = Concatenate Strings(w197, w205, ".msr" ("string")) -> (w203:string)
                n267 = Build Path(base path=w202, name or relative path=w203) -> (appended path=w209:path)
                n268 = Open/Create/Replace File(file path (use dialog)=w209, operation (0:open)=T6."replace or create", access (0:read/write)=enum16{"read/write", "read-only", "write-only"}."write-only") -> (refnum out=w212:refnum<file>)  [unwired: 3 in, 2 out]
                n269 = Concatenate Strings("power" ("string"), w192, "FWHM" ("string"), w192, "peak value" ("string"), w192, "peak location" ("string"), "\r") -> (w189:string)
                n270 = Write to Text File(file (use dialog)=w212, text=w189) -> (refnum out=w196:refnum<file>)  [unwired: 2 in, 2 out]
                n271 = Refnum to Path(1:w196) -> (0:w211:path)
                n272 = call-poly <vilib>:"Write To Spreadsheet File.vi"("transpose? (no:F)"=TRUE, "format (%.3f)"="%6f" ("format string"), "append to file? (new file:F)"=TRUE, "2D data"=w201, "file path (dialog if empty)"=w211) -> ()  [unwired: 3 in, 1 out]
              }
              frame #2 {
                n273 = One Button Dialog(message="Saved !!! ") -> ()  [unwired: 1 in, 1 out]
              }
            }
          }
          frame "Reload Settings", Default {
          }
        }
      }
      n274 = Release Queue(queue=w42, error in (no error)=w41) -> (error out=w43:errorcluster)  [unwired: 1 in, 2 out]
      n275 = call <vilib>:"Simple Error Handler.vi"("error in (no error)"=w43) -> ()  [unwired: 4 in, 5 out]
    }
    frame Error {
    }
  }
  n276 = while {
    tunnel: w5 -> [w556]
    tunnel: w4 -> [_]
    tunnel: [w555] -> w11
    stop <- FALSE stop-if-true
    # "Ocean Optics"
    n277 = global read "GlobalVariables.vi" "SpecDelayreturn"() -> (w540:u32)
    n278 = flat-sequence {
      tunnel: "Average" -> [w561]
      tunnel: "Integration Time" -> [w562]
      tunnel: w556 -> [w563]
      tunnel: "Correct Electrical Dark" -> [w564]
      tunnel: [w564] -> w551
      tunnel: [w563] -> w550
      tunnel: [w562] -> w549
      tunnel: [w561] -> w548
      tunnel: [w560] -> w546
      tunnel: w540 -> [w559]
      tunnel: [w570] -> w552
      tunnel: w551 -> [w573]
      tunnel: w550 -> [w571]
      tunnel: w549 -> [w569]
      tunnel: w548 -> [w568]
      tunnel: w546 -> [w565]
      tunnel: [w565] -> w545
      tunnel: [w577] -> w555
      tunnel: w552 -> [w577]
      tunnel: [w575] -> w541
      tunnel: w545 -> [w574]
      tunnel: [w574] -> w544
      frame #0 {
        n279 = Tick Count (ms)() -> (millisecond timer value=w560:u32)
        n280 = Subtract(x=w560, y=w559) -> (x-y=→"Delayreturn":u32)
      }
      frame #1 {
        n281 = call "Omni-Driver-Fast-Acquire-AVG.vi"("Average"=w568, "Correct Electrical Dark"=w573, "Spectrometer number"=0, "Integration Time (ms)"=w569, "Wrapper"=w571) -> ("Spectrum Values"=w566:dbl[], "WL Values"=w567:dbl[], "Wrapper Out"=w570:u32)  [unwired: 1 out]
        n282 = global write "GlobalVariables.vi" "Wavelenght"(w567) -> ()
        n283 = global write "GlobalVariables.vi" "Spectrum Values"(w566) -> ()
      }
      frame #2 {
        n284 = global write "GlobalVariables.vi" "Spectrum Ready"(TRUE ("Spectrum Ready")) -> ()
        n285 = Tick Count (ms)() -> (millisecond timer value=w575:u32)
      }
    }
    n286 = Subtract(x=w541, y=w544) -> (x-y=→"Spectrum delay (ms)":u32)
    n287 = global write "GlobalVariables.vi" "SpecDelayreturn"(w541) -> ()
    n288 = Wait (ms)(milliseconds to wait=u32 10) -> ()  [unwired: 1 out]
  }
  n289 = while {
    tunnel: w2 -> [w593]
    tunnel: w1 -> [w588]
    tunnel: [w594] -> w14
    tunnel: [w585] -> w13
    stop <- "Stop" stop-if-true
    # "Get Power"
    # "Power Meter"
    n290 = flat-sequence {
      tunnel: w588 -> [w599]
      tunnel: [w599] -> w587
      tunnel: [w598] -> w583
      frame #0 {
        n291 = Tick Count (ms)() -> (millisecond timer value=w598:u32)
      }
    }
    n292 = Wait (ms)(milliseconds to wait=u32 10) -> ()  [unwired: 1 out]
    n293 = call <instrlib>:"TLPM Set Average Time.vi"("error in (no error)"=w587, "Average Time (0.0)"="Average Time (0.0)", "instrument handle"=w593) -> ("error out"=w591:errorcluster, "instrument handle out"=w595:refnum<visa-resource-name>)  [unwired: 7 in]
    n294 = call "TLPM Measure Power.vi"("error in (no error)"=w591, "instrument handle"=w595) -> ("error out"=w589:errorcluster, "Power"=w580:dbl, "instrument handle out"=w594:refnum<visa-resource-name>)  [unwired: 7 in]
    n295 = Divide(x=w580, y="correction factor") -> (x/y=w578:dbl)
    "Power Value" <- w578
    n296 = flat-sequence {
      tunnel: w589 -> [w601]
      tunnel: [w601] -> w586
      frame #0 {
        n297 = global write "GlobalVariables.vi" "Power Meter Ready"(TRUE ("Power Meter Ready")) -> ()
      }
    }
    n298 = global write "GlobalVariables.vi" "Power Meter"(w578) -> ()
    n299 = flat-sequence {
      tunnel: w586 -> [w597]
      tunnel: [w597] -> w585
      tunnel: [w596] -> w584
      frame #0 {
        n300 = Tick Count (ms)() -> (millisecond timer value=w596:u32)
      }
    }
    n301 = Subtract(x=w584, y=w583) -> (x-y=→"P Meter Delay (ms)":u32)
  }
  n302 = call "Omni-Driver-Fast-Close.vi"("Wrapper In"=w11) -> ()  [unwired: 1 in]
  n303 = call "TLPM Close.vi"("error in (no error)"=w13, "instrument handle"=w14) -> ("error out"=w12:errorcluster)  [unwired: 9 in]
  n304 = flat-sequence {
    tunnel: w12 -> [_]
    frame #0 {
      n305 = Stop() -> ()  [unwired: 1 in]
    }
  }
